vi "CC Main.vi"() -> ()   [LabVIEW 2024]
uses:
  typedefs/CC enum Dither Selection.ctl
  typedefs/CC cluster Hardware Config.ctl
  typedefs/CC cluster Device Index.ctl
  Subsystems/SS cluster Command Queues.ctl
  Subsystems/SS typedef Cmd Queue Reference.ctl
  Subsystems/SS typedef cluster Instrument Command Queue Data.ctl
  hk-channel-class/hk-channel-class/HK Table/HK Table.lvclass
  typedefs/CC cluster System Settings.ctl
  Subsystems/SS cluster Data Queue type.ctl
  Subsystems/Subsystem Class CryoServer/Subsystem CryoServer.lvclass
  C:/Development/rimas/RIMAS/Subsystems/Subsystem Class.lvclass
  Subsystems/Detector/Detector.lvclass
  Subsystems/Subsystem Class Filter Wheel/Subsystem Filter Wheel.lvclass
  Subsystems/Subsystem Class Telescope/Subsystem Telescope.lvclass
  Subsystems/Subsystem Class Focus/Subsystem Class Focus.lvclass
  Subsystems/Subsystem CryoCooler/Subsystem CryoCooler.lvclass
  Subsystems/Subsystem Pressure Monitor/Subsystem Pressure Monitor.lvclass
  Subsystems/Subsystem Class Temp Control/Subsystem Class Temp Control.lvclass
  Subsystems/SS cluster Script Status Queue.ctl
  typedefs/CC cluster Observation.ctl
  Observation Queue/CC enum Observation Status.ctl
  Telescope/CC cluster Telescope Offsets.ctl
  typedefs/CC cluster Observation Dither Options.ctl
  typedefs/CC cluster RA and DEC.ctl
  Telescope/Telescope cluster Rotator.ctl
  library/Activity Log/Activity Log enum Action .ctl
  Subsystems/Subsystem Class.lvclass/Subsystem Class.ctl
  typedefs/CC cluster Script.ctl
  typedefs/CC Script Step.ctl
  typedefs/CC enum Script Action.ctl
  Scripts/CC Rd Wr Script Action.ctl
  typedefs/CC enum Alarm Action.ctl
  Logging/CC enum Current Values Action.ctl
  typedefs/CC cluster Script Status Data.ctl
  Subsystems/SS Read cmd q.vi
  54ac6f3e-f790-48ea-ae38-f3b11f920432.vi
  <vilib>/Utility/error.llb/Trim Whitespace One-Sided.vi
  <vilib>/Utility/TDMS File Viewer/TDMS - File Viewer (NXG Style).vi
  <vilib>/Comparison/Less/Less Functor/Less Functor.lvclass
  <vilib>/regexp/Match Regular Expression.xnode
  Subsystems/Subsystem Class.lvclass
  hk-channel-class/hk-channel-class/HK Item/HK Item.lvclass
  <vilib>/Utility/TDMS File Viewer/NI_TDMS File Viewer.lvlib
panel:
  in  "Tab Control":T1(tab)
  in  "Save As Button":bool
  in  "Load":bool
  in  "Get Image":bool
  in  "DEC dither offset":dbl caption="DEC" format="%.1g"
  in  "RA Dither Offset":dbl caption="RA" format="%.1g"
  in  "Filter 4":u16(ring) caption="Slit" items=["pinhole", "1.2'' long", "2.0''", "1.0''", "0.6''", "open"]
  in  "Filter 3":u16(ring) caption="Aux" items=["open", "ND3", "blank", "H2", "2180", "2190", "Br-g"]
  in  "Priority":i32
  in  "Comment":string
  out "Observation File":string
  in  "Block ID":string
  in  "Images":i32=1 min=1 step=1
  in  "Phase":dbl format="%.1g"
  in  "ROT PA":dbl
  in  "eta":dbl
  in  "xi":dbl
  in  "DEC":string
  in  "RA":string
  in  "Obj Type":T2(ring)
  in  "Obj Name":string
  in  "Observer":string
  in  "Add to Q top":bool
  in  "Add to Q":bool
  out "Current DEC":string
  out "Current RA":string
  in  "Replace":bool
  in  "Add Obs Row":bool
  in  "Generate Script":bool
  in  "Save Obs List":bool
  in  "Radius":dbl format="%.1g"
  in  "Int Time":dbl format="%.1g"
  in  "Spots":i32=1 min=1 step=1
  in  "Dither":T3
  in  "Filter 2":u16(ring) caption="FW HK" items=["Grism", "Open", "Vph30", "Vph300", "H", "K"]
  in  "Filter 1":u16(ring) caption="FW YJ" items=["Grism", "Open", "Vph30", "Vph300", "J", "Y"]
  in  "Observation List":i32[](listbox)
  in  "Edit FITS Hdr":bool
  in  "Log 2":bool caption="Log"
  in  "Log":bool
  in  "Export Cryo Data":bool
  out "XY Graph":cluster{timestamp[], dbl[]}[](graph)
  in  "Plot":bool
  in  "Channels":i32[](listbox)
  in  "Open Log":bool
  in  "Note for Log":string
  in  "Send":bool
  in  "Close":bool
  in  "Image Type":u16(ring) items=["raw", "res"]
  in  "Recent Images":i32(listbox)
  out "Status":string
  out "Progress":u8(slide) scale=0.0..100.0
  out "Current File":string
  in  "Data Folder":path
  in  "Clear Alarms":bool
  out "Temp":bool
  out "Cryo Alarm":bool
  out "Pressure Alarm":bool
  out "Telescope Alarm":bool
  out "FW Alarm":bool
  out "Detector Alarm":bool
  out "Alarm Message":string
  out "Alarm Status":bool
  in  "Add offsets":bool
  out "offset (\")":dbl[](array[numeric]) format="%#_3g"
  out "Thumbnail":sgl[][](graph)
  in  "zoom size":i32=20
  out "Zoom":sgl[][](graph)
  out "Console":string
  in  "Tab Control 2":enum32{"Observation Queue", "Slice"}(tab)
  out "Waveform Graph":cluster{"image":sgl[]}[](graph)
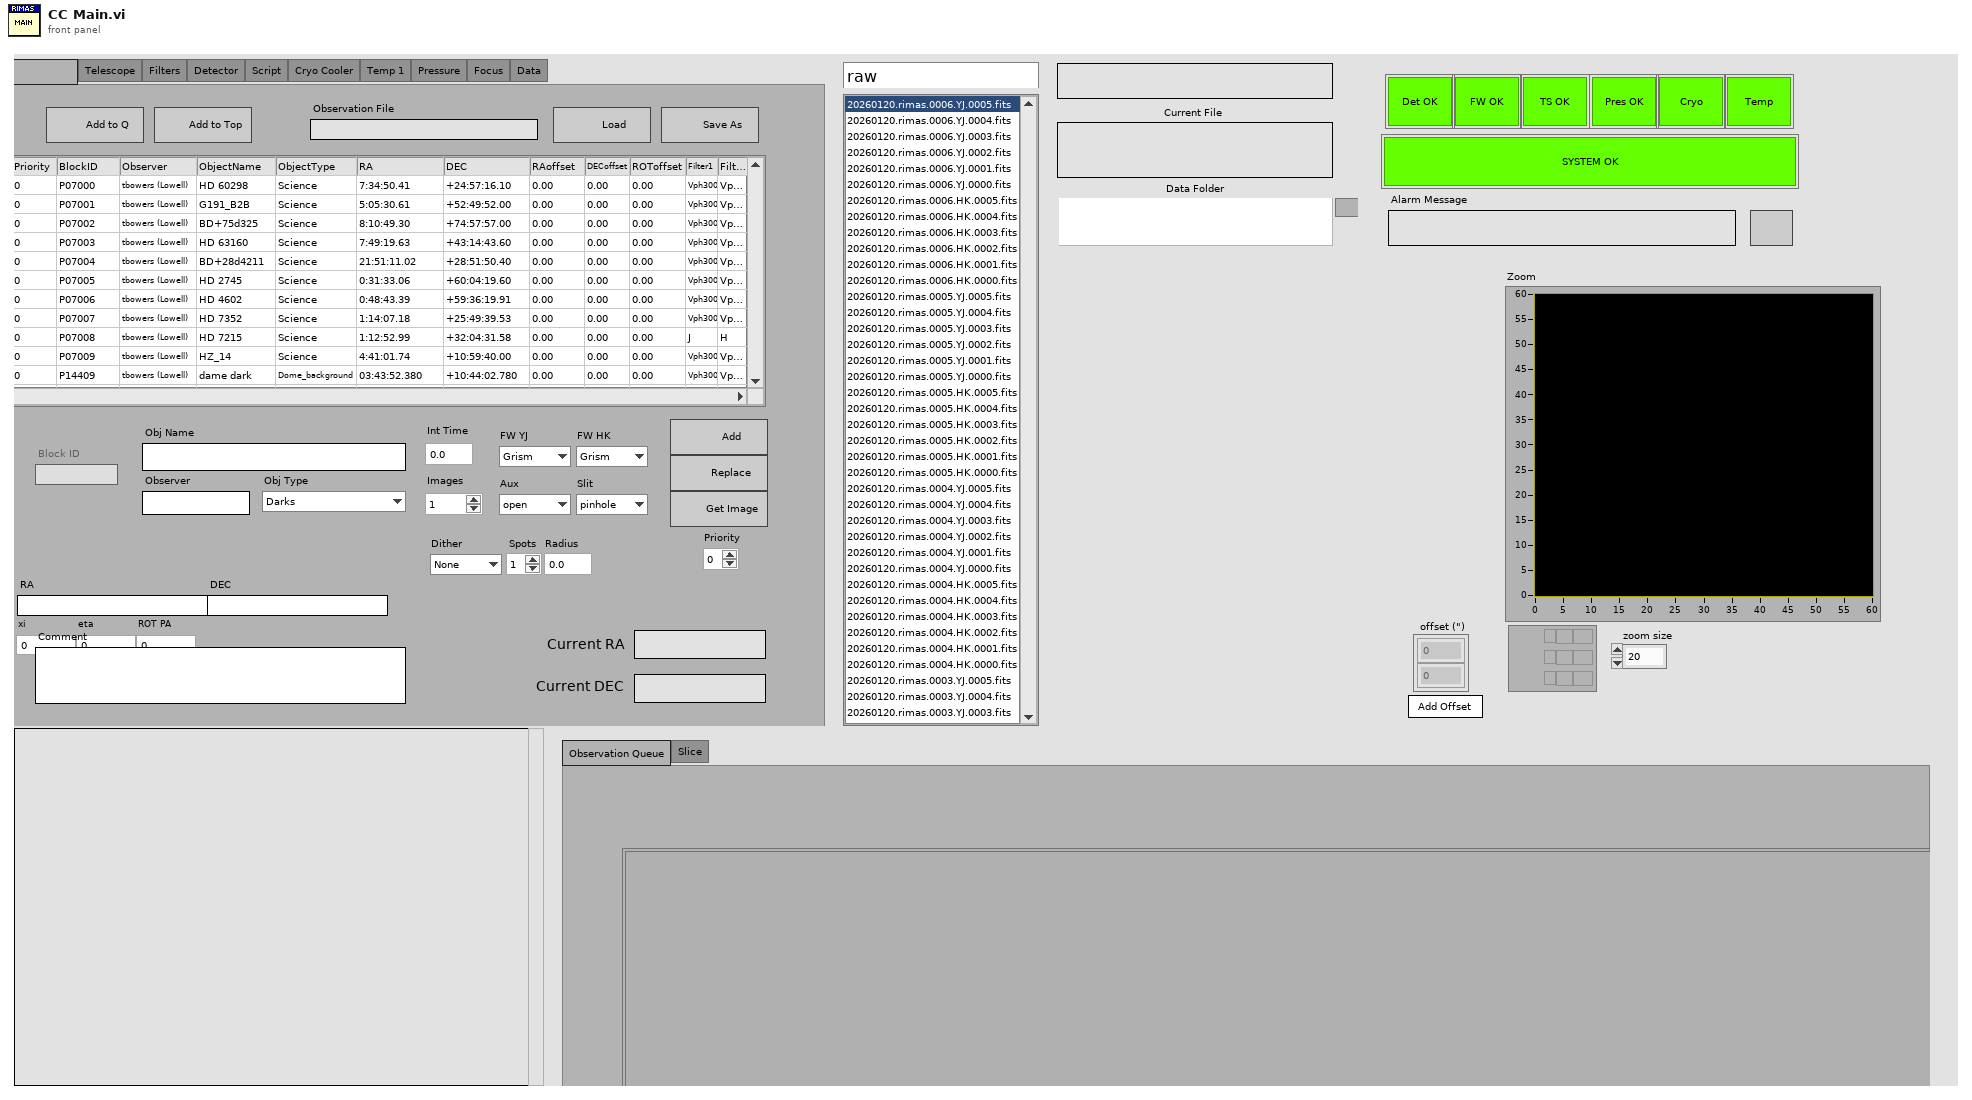
[diagram p1: front panel]
types:
  T1 = enum32{"Observations", "Telescope", "Filters", "Detector", "Script", "Temperatures", "Cryo Cooler", "Temp 1", "Temp 2", "Temp 3", "Pressure", "Focus", "Data"}
  T2 = enum16{"Darks", "Dome_flat", "Sky_flat", "Comparison_lamp", "Comparison_sky", "Dome_background", "Science", "Science_crowded", "Science_extended", "a0v", "Standard", "Tel_focus", "Inst_focus", "Test"}
  T3 = typedef "CC enum Dither Selection.ctl" = enum16{"None", "Circle", "Random", "ABBA", "OnOff"}
  T4 = enum32{"invalid app kind", "Development System", "Run Time System", "Student Edition", "Embedded LabVIEW", "Evaluation", "Custom"}
  T5 = typedef "CC cluster Hardware Config.ctl" = cluster{"Installed Hardware":T6[]}
  T6 = typedef "CC cluster Device Index.ctl" = cluster{"Device Type Name":string, "Curr Device Name":string, "All Instances":string[]}
  T7 = typedef "SS cluster Command Queues.ctl" = cluster{"Telescope Q":T8, "Filter Wheel Q":T8, "Script Q":T8, "CryoServer Q":T8, "Detector Q":T8, "Focus Q":T8, "Temp Ctl 1":T8, "Temp Ctl 2":T8, "Temp Ctl 3":T8, "CryoCooler Q":T8, "Pressure Q":T8}
  T8 = typedef "SS typedef Cmd Queue Reference.ctl" = refnum<queue>
  T9 = typedef "CC cluster System Settings.ctl" = cluster{"HK Table Name":string, "Images Folder":path, "Obs File":path}
  T10 = typedef "CC cluster Observation.ctl" = cluster{"Priority":i32, "ID":string, "Observer":string, "Obj Name":string, "Obj Type":string, "RA and DEC String":cluster{"RA":string, "DEC":string}, "Filters":string[], "Integration Time":dbl, "Observation Status":T11, "Offsets":T12, "Images":i32, "Dither Options":T13, "Comment 1":string, "Comment 2":string, "Rotator":T15}
  T11 = typedef "CC enum Observation Status.ctl" = enum16{"Ready", "Running", "Done", "Error"}
  T12 = typedef "CC cluster Telescope Offsets.ctl" = cluster{"xi":dbl, "eta":dbl, "Offset Type":enum16{"SIMPLE", "TPLANE", "PA"}}
  T13 = typedef "CC cluster Observation Dither Options.ctl" = cluster{"Dither":T3, "Dither Radius":dbl, "Dither Points":i32, "Dither Phase":dbl, "B Offset":T14}
  T14 = typedef "CC cluster RA and DEC.ctl" = cluster{"RA":dbl, "DEC":dbl}
  T15 = typedef "Telescope cluster Rotator.ctl" = cluster{"Frame":enum16{"Target", "Fixed"}, "PA":dbl}
  T16 = cluster{"state":refnum<user-event>, "Hardware":T5, "error":errorcluster, "Cmd Qs":T7, "HK Channels":refnum<class "HK Table.lvclass">, "System Settings":T9, "Data Q":refnum<queue>, "file path":path, "SS":cluster{"CryoServer":refnum<class "Subsystem CryoServer.lvclass">, "Detector":refnum<class "Detector.lvclass">, "Filter Wheel":refnum<class "Subsystem Filter Wheel.lvclass">, "Telescope":refnum<class "Subsystem Telescope.lvclass">, "Focus":refnum<class "Subsystem Class Focus.lvclass">, "CryoCooler":refnum<class "Subsystem CryoCooler.lvclass">, "Pressure":refnum<class "Subsystem Pressure Monitor.lvclass">, "Temp Ctl 1":refnum<class "Subsystem Class Temp Control.lvclass">, "Temp Ctl 2":refnum<class "Subsystem Class Temp Control.lvclass">, "Temp Ctl 3":refnum<class "Subsystem Class Temp Control.lvclass">}, "Script Status Q":refnum<queue>, "Status Data":variant, "curr image":path, "image":sgl[][], "Application:Kind":enum32{"invalid app kind", "Development System", "Run Time System", "Student Edition", "Embedded LabVIEW", "Evaluation", "Custom"}, "Observation List":T10[], "Viewer Ref":refnum<vi>, "Quad Viewer Ref":refnum<vi>, "Obs Queue":refnum<queue>, "Queue vi ref":refnum<vi>, "Script Running":bool, "Wheel Ref":refnum<vi>[], "Observation":T10, "alarm disable":bool, "image types":map{string, path}}
  T17 = typedef "SS cluster Data Queue type.ctl" = cluster{"Source":string, "Type":string, "Data":variant}
  T18 = typedef "Activity Log enum Action .ctl" = enum16{"Add Entry", "Get Log", "Restore From Disk", "Save to Disk", "Init"}
  T19 = typedef "SS typedef cluster Instrument Command Queue Data.ctl" = cluster{"Cmd":string, "Parameters":variant}
  T20 = enum8{"Enabled", "Disabled", "Disabled and Grayed Out"}
  T21 = typedef "CC Rd Wr Script Action.ctl" = enum16{"Read", "Write", "List", "Delete"}
  T22 = typedef "CC cluster Script.ctl" = cluster{"Name":string, "Script":T23[]}
  T23 = typedef "CC Script Step.ctl" = cluster{"Action":T24, "Data":variant}
  T24 = typedef "CC enum Script Action.ctl" = enum16{"Noop", "Define Object", "Define Exposure", "Define Dithering", "Acquire Images", "Set Filter Wheel", "Telescope Home", "Telescope Move", "Telescope RA DEC", "Focus Move Relative", "Focus Move Absolute", "Focus Set Home", "Macro", "Pause", "Ask User", "Define Random Dither", "CmdLine", "Outlet"}
  T25 = typedef "CC enum Alarm Action.ctl" = enum16{"Init", "Add Alarm", "Get Alarms", "Clear Alarm", "Clear All Alarms"}
  T26 = typedef "CC enum Current Values Action.ctl" = enum16{"Init", "Write Item", "Write Array", "Read Item", "Read Array", "Read All", "Add Channels", "New File", "Add Message", "Get Current Values", "Close"}
  T27 = typedef "CC cluster Script Status Data.ctl" = cluster{"Time":timestamp, "Running":bool, "Step":i32, "Script Name":string, "Step Name":string}
  T28 = typedef "SS cluster Script Status Queue.ctl" = cluster{"Msg":string, "Data":variant}
  T29 = typedef "CC cluster Script Panel Defaults.ctl" = cluster{"Script Name":string, "Script Path":path}
  T30 = typedef "CC cluster Alarm Data.ctl" = cluster{"Measured Value":dbl, "Alarm Low":dbl, "Alarm High":dbl, "Message":string, "Source":string}
  T31 = typedef "SS cluster New Image Data.ctl" = cluster{"Frame number":i32, "Detector #":u16, "FITS file":path, "File size":i64, "Image Type":string}
  T32 = typedef "LVCursorListTypeDef.ctl" = cluster{"Name":string, "Color":u32, "Style":u8, "Point Style":u8, "Name Visible":bool, "Allow Drag":bool, "Cursor Mode":u32, "Plot":i32, "Index":i32, "Position":cluster{"X":dbl, "Y":dbl}, "X Scale":u32, "Y Scale":u32, "Watch Plots":i32[], "Watch All Plots":bool, "Plot Area":i32, "Label Offset":cluster{"X":dbl, "Y":dbl}}[]
  T33 = cluster{"Name":string, "Color":u32, "Style":u8, "Point Style":u8, "Name Visible":bool, "Allow Drag":bool, "Cursor Mode":u32, "Plot":i32, "Index":i32, "Position":cluster{"X":dbl, "Y":dbl}, "X Scale":u32, "Y Scale":u32, "Watch Plots":i32[], "Watch All Plots":bool, "Plot Area":i32, "Label Offset":cluster{"X":dbl, "Y":dbl}}
  T34 = cluster{"CryoServer":refnum<class "Subsystem CryoServer.lvclass">, "Detector":refnum<class "Detector.lvclass">, "Filter Wheel":refnum<class "Subsystem Filter Wheel.lvclass">, "Telescope":refnum<class "Subsystem Telescope.lvclass">, "Focus":refnum<class "Subsystem Class Focus.lvclass">, "CryoCooler":refnum<class "Subsystem CryoCooler.lvclass">, "Pressure":refnum<class "Subsystem Pressure Monitor.lvclass">, "Temp Ctl 1":refnum<class "Subsystem Class Temp Control.lvclass">, "Temp Ctl 2":refnum<class "Subsystem Class Temp Control.lvclass">, "Temp Ctl 3":refnum<class "Subsystem Class Temp Control.lvclass">}
  T35 = typedef "LVPoint32TypeDef.ctl" = cluster{"Horizontal":i32, "Vertical":i32}
  T36 = typedef "LVRowAndColumnTypeDef.ctl" = cluster{"Row":i32, "Column":i32}
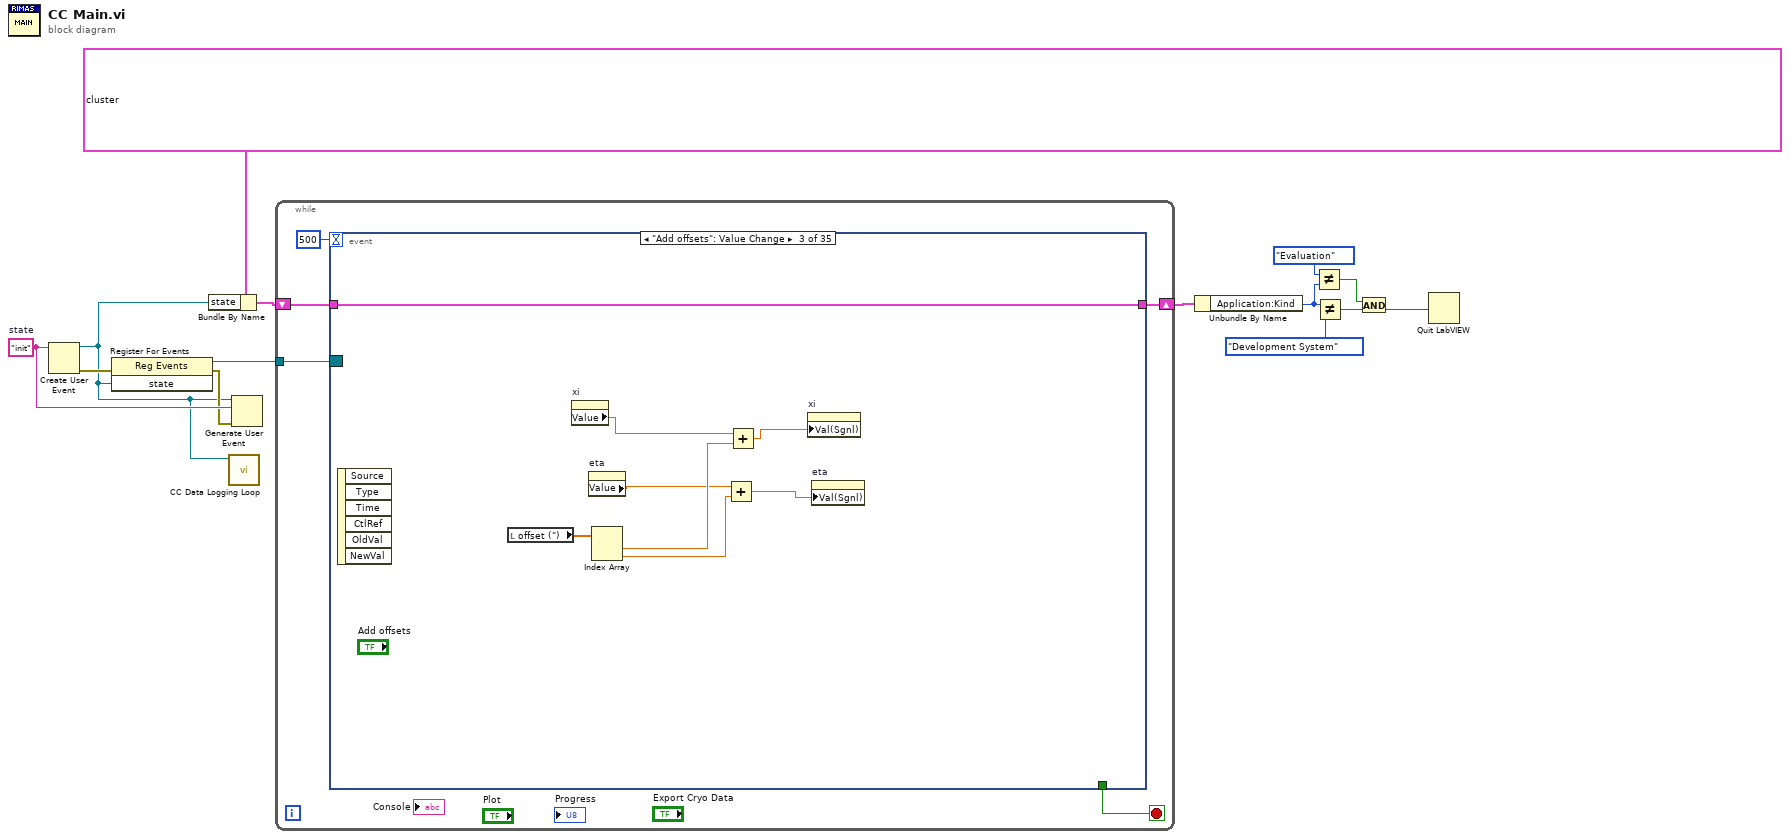
[diagram p0: block diagram]
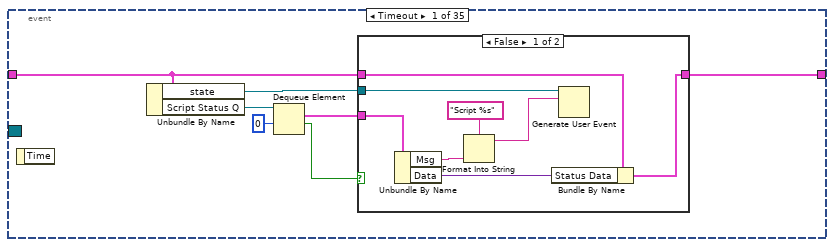
[diagram p2: hidden frame]
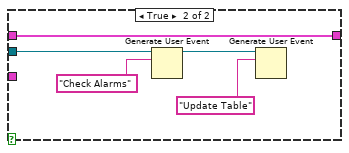
[diagram p3: hidden frame]
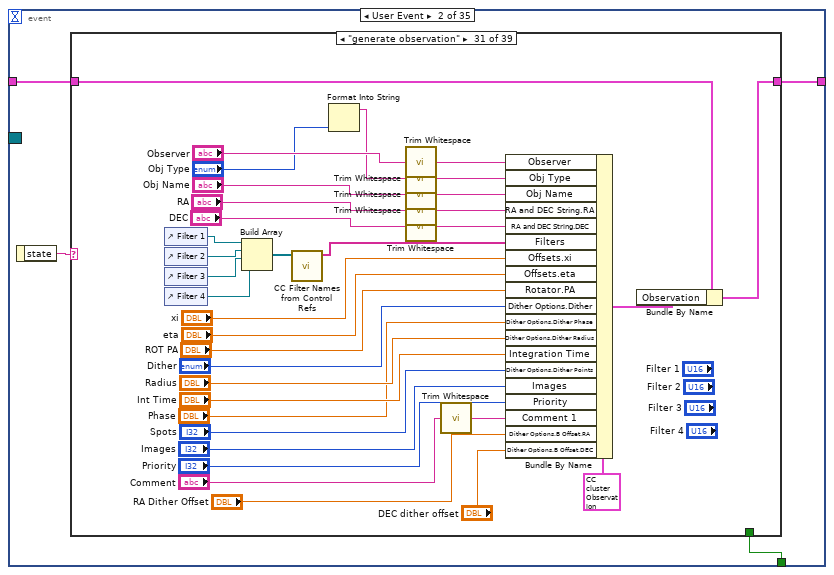
[diagram p4: hidden frame]
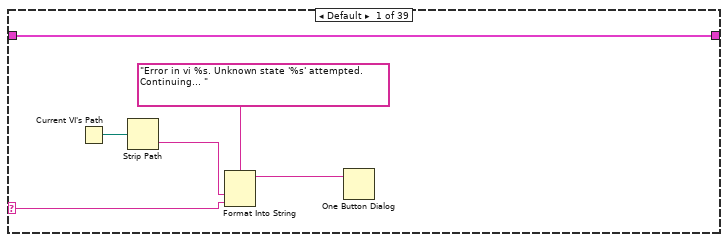
[diagram p5: hidden frame]
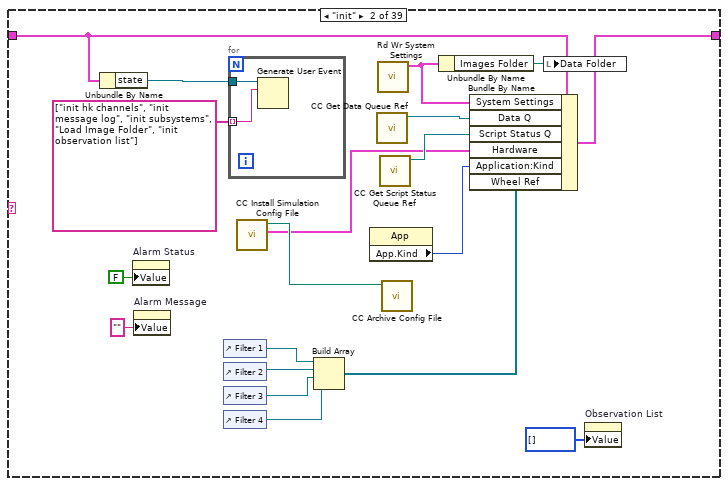
[diagram p6: hidden frame]
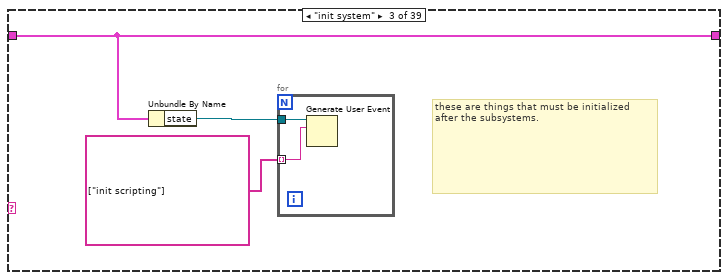
[diagram p7: hidden frame]
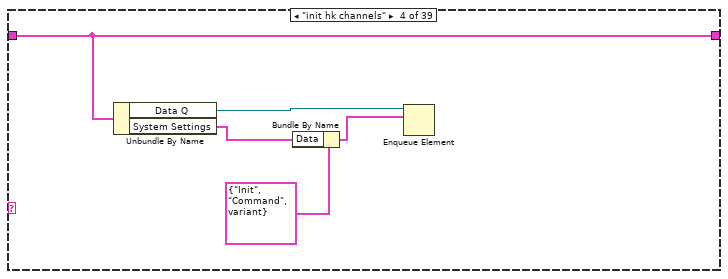
[diagram p8: hidden frame]
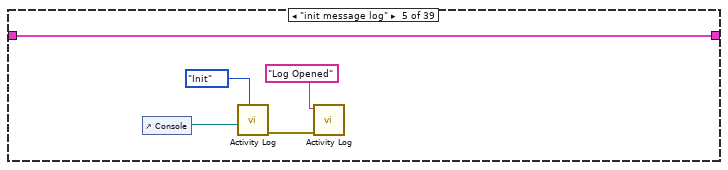
[diagram p9: hidden frame]
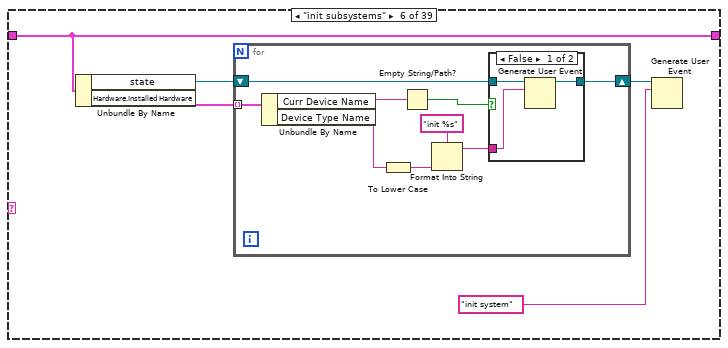
[diagram p10: hidden frame]
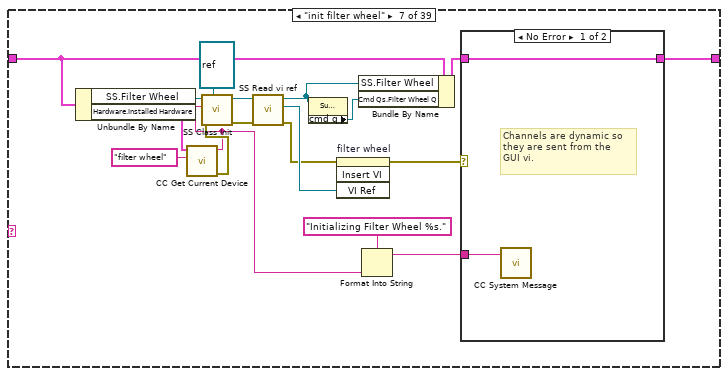
[diagram p12: hidden frame]
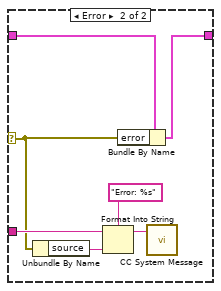
[diagram p13: hidden frame]
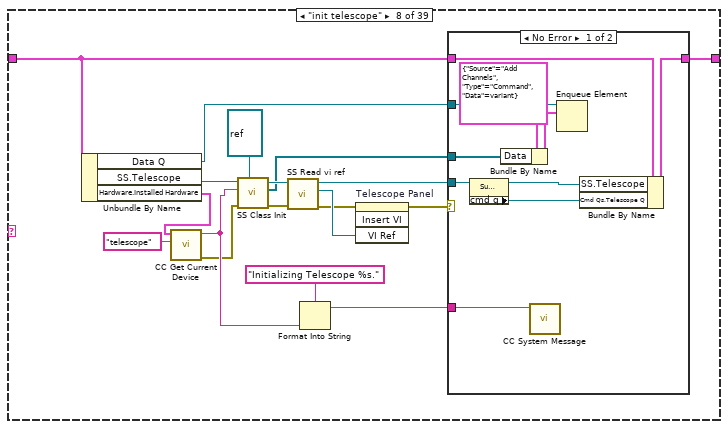
[diagram p14: hidden frame]
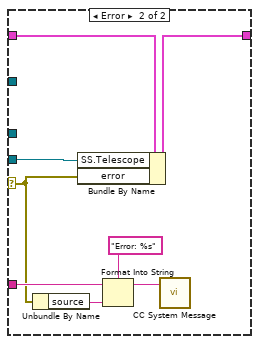
[diagram p15: hidden frame]
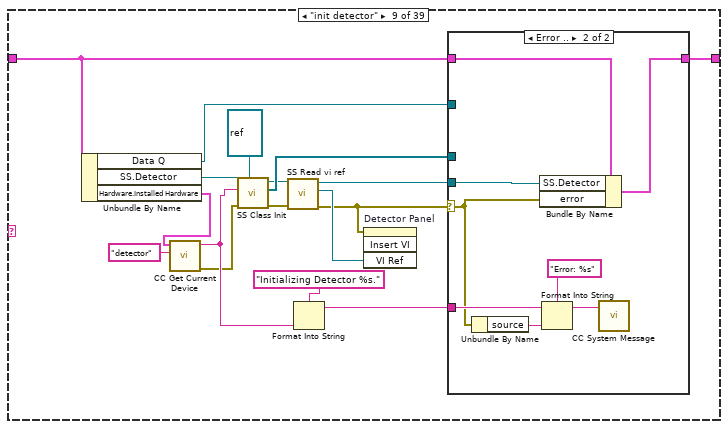
[diagram p16: hidden frame]
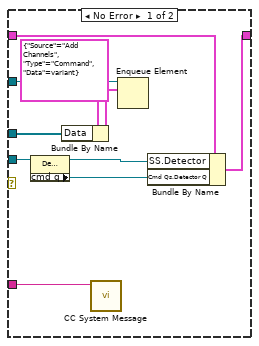
[diagram p17: hidden frame]
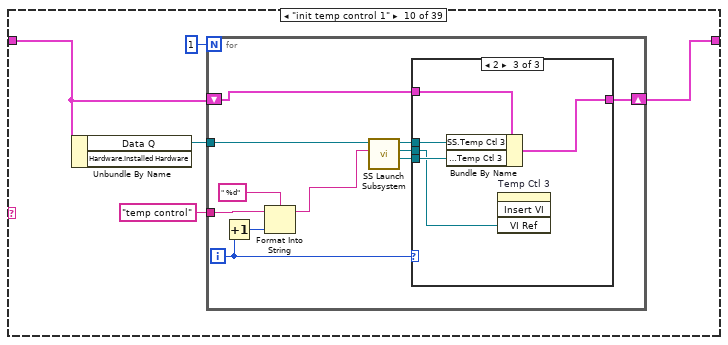
[diagram p18: hidden frame]
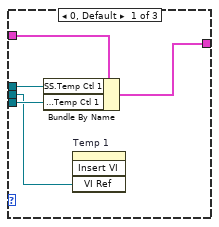
[diagram p19: hidden frame]
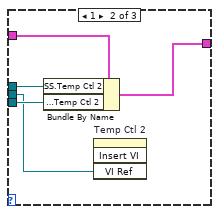
[diagram p20: hidden frame]
diagram:
  w11 = "init"  # state
  n1 = Create User Event(user event datatype=w11) -> (user event=w8:refnum<user-event>, error out=w9:errorcluster)  [unwired: 1 in]
  n2 = register-events(error in=w9, w8) -> (reference out=w12:refnum<event-registration>, error out=w10:errorcluster)  [unwired: 1 in]
  n3 = Bundle By Name(cluster=T16 {"state"=refnum, "Hardware"={"Installed Hardware"=[]}, "error"={"status"=FALSE, "code"=0, "source"=""}, "Cmd Qs"={"Telescope Q"=refnum, "Filter Wheel Q"=refnum, "Script Q"=refnum, "CryoServer Q"=refnum, "Detector Q"=refnum, "Focus Q"=refnum, "Temp Ctl 1"=refnum, "Temp Ctl 2"=refnum, "Temp Ctl 3"=refnum, "CryoCooler Q"=refnum, "Pressure Q"=refnum}, "HK Channels"=refnum, "System Settings"={"HK Table Name"="", "Images Folder"=path "", "Obs File"=path ""}, "Data Q"=refnum, "file path"=path "", "SS"={"CryoServer"=refnum, "Detector"=refnum, "Filter Wheel"=refnum, "Telescope"=refnum, "Focus"=refnum, "CryoCooler"=refnum, "Pressure"=refnum, "Temp Ctl 1"=refnum, "Temp Ctl 2"=refnum, "Temp Ctl 3"=refnum}, "Script Status Q"=refnum, "Status Data"=variant, "curr image"=path "", "image"=[], "Application:Kind"=enum."invalid app kind", "Observation List"=[], "Viewer Ref"=refnum, "Quad Viewer Ref"=refnum, "Obs Queue"=refnum, "Queue vi ref"=refnum, "Script Running"=FALSE, "Wheel Ref"=[], "Observation"={"Priority"=0, "ID"="", "Observer"="", "Obj Name"="", "Obj Type"="", "RA and DEC String"={"RA"="12:34:56.789", "DEC"="010:11:12.013"}, "Filters"=[], "Integration Time"=0.0, "Observation Status"=enum."Ready", "Offsets"={"xi"=0.0, "eta"=0.0, "Offset Type"=enum."SIMPLE"}, "Images"=0, "Dither Options"={"Dither"=enum."None", "Dither Radius"=0.0, "Dither Points"=0, "Dither Phase"=0.0, "B Offset"={"RA"=0.0, "DEC"=0.0}}, "Comment 1"="", "Comment 2"="", "Rotator"={"Frame"=enum."Target", "PA"=0.0}}, "alarm disable"=FALSE, "image types"={}}, "state"=w8) -> (w13:T16)
  n4 = call "CC Data Logging Loop.vi"("user event"=w8) -> ()  [unwired: 11 in]
  n5 = Generate User Event(user event=w8, event data cluster=w11, error in=w10) -> ()  [unwired: 1 in, 2 out]
  n6 = while {
    tunnel: w12 -> [w19]
    shift-right: [w17] -> w7
    shift-left: w13 -> [w18]
    stop <- w16 stop-if-true
    n7 = event shown="[2] \"Add offsets\": Value Change" {
      selector: w19 -> [_ _ _ _ _ _ _ _ _ _ _ _ _ _ _ _ _ _ _ _ _ _ _ _ _ _ _ _ _ _ _ _ _ _ _]
      dyn-events: _ -> [_ _ _ _ _ _ _ _ _ _ _ _ _ _ _ _ _ _ _ _ _ _ _ _ _ _ _ _ _ _ _ _ _ _ _]
      timeout: 500 -> [_ _ _ _ _ _ _ _ _ _ _ _ _ _ _ _ _ _ _ _ _ _ _ _ _ _ _ _ _ _ _ _ _ _ _]
      tunnel: w18 -> [w24 w42 w809 w812 w878 w881 w917 w919 w924 w954 w985 w991 w1011 w1019 w1022 w1027 w1033 w1039 w1042 w1044 w1051 w1189 w1202 w1219 w1222 w1225 w1227 w1230 w1236 w1237 w1245 w1259 w1263 w1270 w1276]
      tunnel: [w21 w41 w809 w811 w878 w881 w917 w919 w926 w954 w985 w992 w1011 w1019 w1022 w1027 w1033 w1039 w1042 w1044 w1052 w1189 w1204 w1219 w1222 w1225 w1227 w1230 w1236 w1237 w1241 w1259 w1263 w1267 w1276] -> w17
      tunnel: [_ w40 _ _ _ _ _ _ _ _ _ _ _ _ _ _ _ _ _ _ _ _ _ _ _ _ _ _ FALSE ("Close") _ _ _ _ _ _] -> w16
      event Timeout {
        n8 = event-data() -> ()  [unwired: 1 in, 1 out]
        n9 = Unbundle By Name(w24) -> ("state"=w23:refnum<user-event>, "Script Status Q"=w26:refnum<queue>)
        n10 = Dequeue Element(queue=w26, timeout in ms (-1)=0) -> (element=w22:T28, timed out?=w25:bool)  [unwired: 1 in, 2 out]
        n11 = case shown="False" w25 {
          tunnel: w24 -> [w29 w39]
          tunnel: w23 -> [w34 w38]
          tunnel: w22 -> [w33 _]
          tunnel: [w27 w39] -> w21
          frame False {
            n12 = Unbundle By Name(w33) -> ("Msg"=w31:string, "Data"=w28:variant)
            n13 = Format Into String(format string="Script %s", w31) -> (resulting string=w30:string)  [unwired: 2 in, 1 out]
            n14 = Bundle By Name(cluster=w29, "Status Data"=w28) -> (w27:T16)
            n15 = Generate User Event(user event=w34, event data cluster=w30) -> ()  [unwired: 2 in, 2 out]
          }
          frame True {
            n16 = Generate User Event(user event=w38, event data cluster="Check Alarms" ("event data")) -> (user event out=w36:refnum<user-event>)  [unwired: 2 in, 1 out]
            n17 = Generate User Event(user event=w36, event data cluster="Update Table" ("event data")) -> ()  [unwired: 2 in, 2 out]
          }
        }
      }
      event User Event {
        n18 = event-data() -> ("state"=w43:string)  [unwired: 1 in]
        n19 = case shown="\"generate observation\"" w43 {
          selector: w43 -> [w48 _ _ _ _ _ _ _ _ _ _ _ _ _ _ _ _ _ _ _ _ _ _ _ _ _ _ _ _ _ _ _ _ _ _ _ _ _ _]
          tunnel: w42 -> [w44 w65 w72 w76 w85 w90 w114 w144 w181 w204 w233 w244 w276 w307 w342 w364 w395 w404 w419 w437 w446 w453 w478 w497 w542 w568 w598 w616 w656 w663 w675 w706 w713 w721 w725 w770 w773 w782 w792]
          tunnel: [w44 w66 w72 w76 w85 w90 w115 w145 w182 w203 w233 w245 w277 w308 w343 w365 w396 w405 w418 w437 w446 w453 w478 w498 w542 w568 w599 w617 w656 w664 w676 w706 w713 w722 w726 w770 w773 w782 w792] -> w41
          tunnel: [_ _ _ _ _ _ _ _ _ _ _ _ _ _ _ _ _ _ _ _ _ _ _ _ _ _ _ _ _ _ _ _ _ _ _ _ _ FALSE TRUE] -> w40
          frame Default {
            n20 = Current VI's Path() -> (path=w47:path)
            n21 = Strip Path(path=w47) -> (name=w46:string)  [unwired: 1 out]
            n22 = Format Into String(format string="Error in vi %s. Unknown state '%s' attempted. Continuing... ", w46, w48) -> (resulting string=w45:string)  [unwired: 2 in, 1 out]
            n23 = One Button Dialog(message=w45) -> ()  [unwired: 1 in, 1 out]
          }
          frame "init" {
            n24 = Unbundle By Name(w65) -> ("state"=w68:refnum<user-event>)
            n25 = property on="Alarm Status" class="Bool (strict)"("Value"=FALSE ("Alarm Status")) -> ()  [unwired: 2 in, 2 out]
            n26 = property on="Alarm Message" class="Str"("Value"="" ("Alarm Message")) -> ()  [unwired: 2 in, 2 out]
            n27 = control-ref of="Filter 1"() -> (w56:refnum<vi>)
            n28 = control-ref of="Filter 2"() -> (w55:refnum<vi>)
            n29 = control-ref of="Filter 3"() -> (w54:refnum<vi>)
            n30 = control-ref of="Filter 4"() -> (w53:refnum<vi>)
            n31 = for {
              tunnel: w68 -> [w70]
              tunnel: string[] ["init hk channels", "init message log", "init subsystems", "Load Image Folder", "init observation list"] -> [w69] mode=indexing
              n32 = Generate User Event(user event=w70, event data cluster=w69) -> ()  [unwired: 2 in, 2 out]
            }
            n33 = call "CC Install Simulation Config File.vi"() -> ("Hardware Config out"=w50:T5, "new path"=w51:path)  [unwired: 10 in]
            n34 = Build Array(w56, w55, w54, w53) -> (w52:refnum<vi>[])
            n35 = property class="App"() -> ("App.Kind"=w60:T4)  [unwired: 2 in, 2 out]
            n36 = call "CC Get Data Queue Ref.vi"() -> ("Data Q"=w64:refnum<queue>)  [unwired: 10 in, 1 out]
            n37 = call "Rd Wr System Settings.vi"() -> ("System Settings out"=w62:T9)  [unwired: 10 in, 1 out]
            n38 = call "CC Get Script Status Queue Ref.vi"() -> ("Script Status Q"=w63:refnum<queue>)  [unwired: 10 in, 1 out]
            n39 = call "CC Archive Config File.vi"("config file"=w51) -> ()  [unwired: 10 in, 1 out]
            n40 = Unbundle By Name(w62) -> ("Images Folder"=w61:path)
            n41 = Bundle By Name(cluster=w65, "System Settings"=w62, "Data Q"=w64, "Script Status Q"=w63, "Hardware"=w50, "Application:Kind"=w60, "Wheel Ref"=w52) -> (w66:T16)
            n42 = local write "Data Folder"(w61) -> ()
            n43 = property on="Observation List" class="MCListbox (strict)"("Value"=i32[] [] ("Observation List")) -> ()  [unwired: 2 in, 2 out]
          }
          frame "init system" {
            # "these are things that must be initialized after the subsystems."
            n44 = Unbundle By Name(w72) -> ("state"=w73:refnum<user-event>)
            n45 = for {
              tunnel: w73 -> [w75]
              tunnel: string[] ["init scripting"] -> [w74] mode=indexing
              n46 = Generate User Event(user event=w75, event data cluster=w74) -> ()  [unwired: 2 in, 2 out]
            }
          }
          frame "init hk channels" {
            n47 = Unbundle By Name(w76) -> ("Data Q"=w80:refnum<queue>, "System Settings"=w78:T9)
            n48 = Bundle By Name(cluster=T17 {"Source"="Init", "Type"="Command", "Data"=variant} ("element"), "Data"=w78) -> (w77:T17)
            n49 = Enqueue Element(queue=w80, element=w77) -> ()  [unwired: 2 in, 3 out]
          }
          frame "init message log" {
            n50 = control-ref of="Console"() -> (w83:refnum<vi>)
            n51 = call "Activity Log.vi"("Action"=Activity_Log_enum_Action_."Init", "string ref"=w83) -> ("Error Out"=w82:errorcluster)  [unwired: 8 in, 1 out]
            n52 = call "Activity Log.vi"("Error In"=w82, "Message Log Entry"="Log Opened") -> ()  [unwired: 8 in, 2 out]
          }
          frame "init subsystems" {
            n53 = Unbundle By Name(w90) -> ("state"=w89:refnum<user-event>, "Hardware.Installed Hardware"=w88:T6[])
            n54 = for {
              tunnel: w88 -> [w97] mode=indexing
              shift-right: [w91] -> w87
              shift-left: w89 -> [w98]
              n55 = Unbundle By Name(w97) -> ("Curr Device Name"=w93:string, "Device Type Name"=w92:string)
              n56 = To Lower Case(string=w92) -> (all lower case string=w94:string)
              n57 = Empty String/Path?(string/path=w93) -> (empty?=w99:bool)
              n58 = Format Into String(format string="init %s", w94) -> (resulting string=w96:string)  [unwired: 2 in, 1 out]
              n59 = case shown="False" w99 {
                tunnel: w98 -> [w102 w103]
                tunnel: w96 -> [w101 _]
                tunnel: [w100 w103] -> w91
                frame False {
                  n60 = Generate User Event(user event=w102, event data cluster=w101) -> (user event out=w100:refnum<user-event>)  [unwired: 2 in, 1 out]
                }
                frame True {
                }
              }
            }
            n61 = Generate User Event(user event=w87, event data cluster="init system" ("format string")) -> ()  [unwired: 2 in, 2 out]
          }
          frame "init filter wheel" {
            n62 = Unbundle By Name(w114) -> ("SS.Filter Wheel"=w113:refnum<class "Subsystem Filter Wheel.lvclass">, "Hardware.Installed Hardware"=w107:T6[])
            n63 = call "CC Get Current Device.vi"("Device Type Name"="filter wheel", "Hardware.Installed Hardware"=w107) -> ("error out"=w105:errorcluster, "Curr Device Name"=w104:string)  [unwired: 7 in, 1 out]
            n64 = call-dynamic "SS Class Init.vi"("VI Refnum"=refnum<vi> refnum, "error in (no error)"=w105, "Device"=w104, "Subsystem Filter Wheel in"=w113) -> ("error out"=w109:errorcluster, "Subsystem Filter Wheel out"=w112:refnum<class "Subsystem Filter Wheel.lvclass">)  [unwired: 5 in, 1 out]
            n65 = call "SS Read vi ref.vi"("error in (no error)"=w109, "Subsystem Class in"=w112) -> ("error out"=w120:errorcluster, "vi ref"=w121:refnum<vi>, "Subsystem Class out"=w111:refnum<class "Subsystem Filter Wheel.lvclass">)  [unwired: 7 in]
            n66 = property class="Subsystem Filter Wheel.lvclass"(reference=w111) -> ("cmd q"=w110:T8)  [unwired: 1 in, 2 out]
            n67 = invoke on="filter wheel" class="SubPnl" method="Insert VI"(error in=w120, "VI Ref"=w121) -> (error out=w118:errorcluster)  [unwired: 2 in, 3 out]
            n68 = Bundle By Name(cluster=w114, "SS.Filter Wheel"=w111, "Cmd Qs.Filter Wheel Q"=w110) -> (w116:T16)
            n69 = Format Into String(format string="Initializing Filter Wheel %s.", w104) -> (resulting string=w117:string)  [unwired: 2 in, 1 out]
            n70 = case shown="No Error" w118 {
              selector: w118 -> [_ w126]
              tunnel: w117 -> [w123 w127]
              tunnel: w116 -> [w122 w130]
              tunnel: [w122 w129] -> w115
              frame No Error {
                # "Channels are dynamic so\nthey are sent from the \nGUI vi."
                n71 = call "CC System Message.vi"("Message"=w123) -> ()  [unwired: 10 in, 1 out]
              }
              frame Error {
                n72 = Unbundle By Name(w126) -> ("source"=w125:string)
                n73 = Format Into String(format string="Error: %s", initial string=w127, w125) -> (resulting string=w124:string)  [unwired: 1 in, 1 out]
                n74 = Bundle By Name(cluster=w130, "error"=w126) -> (w129:T16)
                n75 = call "CC System Message.vi"("Message"=w124) -> ()  [unwired: 10 in, 1 out]
              }
            }
          }
          frame "init telescope" {
            n76 = Unbundle By Name(w144) -> ("Data Q"=w136:refnum<queue>, "SS.Telescope"=w148:refnum<class "Subsystem Telescope.lvclass">, "Hardware.Installed Hardware"=w133:T6[])
            n77 = call "CC Get Current Device.vi"("Device Type Name"="telescope", "Hardware.Installed Hardware"=w133) -> ("error out"=w131:errorcluster, "Curr Device Name"=w132:string)  [unwired: 7 in, 1 out]
            n78 = call-dynamic "SS Class Init.vi"("VI Refnum"=refnum<vi> refnum, "error in (no error)"=w131, "Device"=w132, "Telescope in"=w148) -> ("error out"=w146:errorcluster, "Channel List"=w137:refnum<class "HK Item.lvclass">[], "Telescope out"=w147:refnum<class "Subsystem Telescope.lvclass">)  [unwired: 5 in]
            n79 = call "SS Read vi ref.vi"("error in (no error)"=w146, "Subsystem Class in"=w147) -> ("error out"=w139:errorcluster, "vi ref"=w140:refnum<vi>, "Subsystem Class out"=w141:refnum<class "Subsystem Telescope.lvclass">)  [unwired: 7 in]
            n80 = Format Into String(format string="Initializing Telescope %s.", w132) -> (resulting string=w142:string)  [unwired: 2 in, 1 out]
            n81 = invoke on="Telescope Panel" class="SubPnl" method="Insert VI"(error in=w139, "VI Ref"=w140) -> (error out=w138:errorcluster)  [unwired: 2 in, 3 out]
            n82 = case shown="No Error" w138 {
              selector: w138 -> [_ w162]
              tunnel: w142 -> [w149 w163]
              tunnel: w144 -> [w155 w166]
              tunnel: [w156 w165] -> w145
              tunnel: w141 -> [w158 w160]
              tunnel: w137 -> [w151 _]
              tunnel: w136 -> [w153 _]
              frame No Error {
                n83 = property class="Subsystem Telescope.lvclass"(reference=w158) -> (reference out=w154:refnum<class "Subsystem Telescope.lvclass">, "cmd q"=w157:T8)  [unwired: 1 in, 1 out]
                n84 = Bundle By Name(cluster=T17 {"Source"="Add Channels", "Type"="Command", "Data"=variant} ("element"), "Data"=w151) -> (w150:T17)
                n85 = call "CC System Message.vi"("Message"=w149) -> ()  [unwired: 10 in, 1 out]
                n86 = Enqueue Element(queue=w153, element=w150) -> ()  [unwired: 2 in, 3 out]
                n87 = Bundle By Name(cluster=w155, "SS.Telescope"=w154, "Cmd Qs.Telescope Q"=w157) -> (w156:T16)
              }
              frame Error {
                n88 = Unbundle By Name(w162) -> ("source"=w161:string)
                n89 = Bundle By Name(cluster=w166, "SS.Telescope"=w160, "error"=w162) -> (w165:T16)
                n90 = Format Into String(format string="Error: %s", initial string=w163, w161) -> (resulting string=w159:string)  [unwired: 1 in, 1 out]
                n91 = call "CC System Message.vi"("Message"=w159) -> ()  [unwired: 10 in, 1 out]
              }
            }
          }
          frame "init detector" {
            n92 = Unbundle By Name(w181) -> ("Data Q"=w176:refnum<queue>, "SS.Detector"=w174:refnum<class "Detector.lvclass">, "Hardware.Installed Hardware"=w171:T6[])
            n93 = call "CC Get Current Device.vi"("Device Type Name"="detector", "Hardware.Installed Hardware"=w171) -> ("error out"=w169:errorcluster, "Curr Device Name"=w170:string)  [unwired: 7 in, 1 out]
            n94 = call-dynamic "SS Class Init.vi"("VI Refnum"=refnum<vi> refnum, "error in (no error)"=w169, "Device"=w170, "Detector in"=w174) -> ("error out"=w183:errorcluster, "Channel List"=w177:refnum<class "HK Item.lvclass">[], "Detector out"=w173:refnum<class "Detector.lvclass">)  [unwired: 5 in]
            n95 = call "SS Read vi ref.vi"("error in (no error)"=w183, "Subsystem Class in"=w173) -> ("error out"=w167:errorcluster, "vi ref"=w168:refnum<vi>, "Subsystem Class out"=w178:refnum<class "Detector.lvclass">)  [unwired: 7 in]
            n96 = Format Into String(format string="Initializing Detector %s.", w170) -> (resulting string=w179:string)  [unwired: 2 in, 1 out]
            n97 = invoke on="Detector Panel" class="SubPnl" method="Insert VI"(error in=w167, "VI Ref"=w168) -> ()  [unwired: 2 in, 4 out]
            n98 = case shown="Error .." w167 {
              selector: w167 -> [_ w197]
              tunnel: w179 -> [w184 w198]
              tunnel: w181 -> [w190 w201]
              tunnel: [w191 w200] -> w182
              tunnel: w178 -> [w193 w195]
              tunnel: w177 -> [w186 _]
              tunnel: w176 -> [w188 _]
              frame No Error {
                n99 = property class="Detector.lvclass"(reference=w193) -> (reference out=w189:refnum<class "Detector.lvclass">, "cmd q"=w192:T8)  [unwired: 1 in, 1 out]
                n100 = Bundle By Name(cluster=T17 {"Source"="Add Channels", "Type"="Command", "Data"=variant} ("element"), "Data"=w186) -> (w185:T17)
                n101 = call "CC System Message.vi"("Message"=w184) -> ()  [unwired: 10 in, 1 out]
                n102 = Enqueue Element(queue=w188, element=w185) -> ()  [unwired: 2 in, 3 out]
                n103 = Bundle By Name(cluster=w190, "SS.Detector"=w189, "Cmd Qs.Detector Q"=w192) -> (w191:T16)
              }
              frame Error {
                n104 = Unbundle By Name(w197) -> ("source"=w196:string)
                n105 = Bundle By Name(cluster=w201, "SS.Detector"=w195, "error"=w197) -> (w200:T16)
                n106 = Format Into String(format string="Error: %s", initial string=w198, w196) -> (resulting string=w194:string)  [unwired: 1 in, 1 out]
                n107 = call "CC System Message.vi"("Message"=w194) -> ()  [unwired: 10 in, 1 out]
              }
            }
          }
          frame "init temp control 1" {
            n108 = Unbundle By Name(w204) -> ("Data Q"=w206:refnum<queue>)  [unwired: 1 out]
            n109 = for {
              N: 1 -> [_]
              tunnel: w206 -> [w217]
              tunnel: "temp control" ("Device Type Name") -> [w214]
              shift-right: [w209] -> w203
              shift-left: w204 -> [w211]
              i -> [w213]
              n110 = Increment(x=w213) -> (x+1=w212:i32)
              n111 = Format Into String(format string=" %d", initial string=w214, w212) -> (resulting string=w207:string)  [unwired: 1 in, 1 out]
              n112 = call "SS Launch Subsystem.vi"("Curr Device Name"=w207, "Data Q"=w217) -> ("cmd q"=w208:T8, "vi ref"=w216:refnum<vi>, "Temp Ctl Class"=w210:refnum<class "Subsystem Class Temp Control.lvclass">)  [unwired: 6 in, 1 out]
              n113 = case shown="2" w213 {
                tunnel: w216 -> [w218 w223 w228]
                tunnel: w211 -> [w222 w227 w232]
                tunnel: w210 -> [w221 w226 w231]
                tunnel: [w220 w225 w230] -> w209
                tunnel: w208 -> [w219 w224 w229]
                frame 0, Default {
                  n114 = Bundle By Name(cluster=w222, "SS.Temp Ctl 1"=w221, "Cmd Qs.Temp Ctl 1"=w219) -> (w220:T16)
                  n115 = invoke on="Temp 1" class="SubPnl" method="Insert VI"("VI Ref"=w218) -> ()  [unwired: 3 in, 4 out]
                }
                frame 1 {
                  n116 = Bundle By Name(cluster=w227, "SS.Temp Ctl 2"=w226, "Cmd Qs.Temp Ctl 2"=w224) -> (w225:T16)
                  n117 = invoke on="Temp Ctl 2" class="SubPnl" method="Insert VI"("VI Ref"=w223) -> ()  [unwired: 3 in, 4 out]
                }
                frame 2 {
                  n118 = Bundle By Name(cluster=w232, "SS.Temp Ctl 3"=w231, "Cmd Qs.Temp Ctl 3"=w229) -> (w230:T16)
                  n119 = invoke on="Temp Ctl 3" class="SubPnl" method="Insert VI"("VI Ref"=w228) -> ()  [unwired: 3 in, 4 out]
                }
              }
            }
          }
          frame "init temp control 2", "init temp control 3" {
          }
          frame "init cryoserver" {
            n120 = Unbundle By Name(w244) -> ("SS.CryoServer"=w248:refnum<class "Subsystem CryoServer.lvclass">, "Hardware.Installed Hardware"=w237:T6[])
            n121 = call "CC Get Current Device.vi"("Device Type Name"="cryoserver", "Hardware.Installed Hardware"=w237) -> ("error out"=w235:errorcluster, "Curr Device Name"=w236:string)  [unwired: 7 in, 1 out]
            n122 = call-dynamic "SS Class Init.vi"("VI Refnum"=refnum<vi> refnum, "error in (no error)"=w235, "Device"=w236, "Subsystem CryoServer in"=w248) -> ("error out"=w246:errorcluster, "Subsystem CryoServer out"=w247:refnum<class "Subsystem CryoServer.lvclass">)  [unwired: 5 in, 1 out]
            n123 = call "SS Read vi ref.vi"("error in (no error)"=w246, "Subsystem Class in"=w247) -> ("error out"=w234:errorcluster, "vi ref"=w239:refnum<vi>, "Subsystem Class out"=w241:refnum<class "Subsystem CryoServer.lvclass">)  [unwired: 7 in]
            n124 = Format Into String(format string="Initializing CryoServer %s.", w236) -> (resulting string=w242:string)  [unwired: 2 in, 1 out]
            n125 = invoke on="Cryo Panel" class="SubPnl" method="Insert VI"("VI Ref"=w239) -> ()  [unwired: 3 in, 4 out]
            n126 = case shown="Error .." w234 {
              selector: w234 -> [_ w258]
              tunnel: w242 -> [w249 w259]
              tunnel: w244 -> [w251 w262]
              tunnel: [w252 w261] -> w245
              tunnel: w241 -> [w254 w256]
              frame No Error {
                # "Note: All Cryo Channels are dynamic\nso no add channels here."
                n127 = property class="Subsystem CryoServer.lvclass"(reference=w254) -> (reference out=w250:refnum<class "Subsystem CryoServer.lvclass">, "cmd q"=w253:T8)  [unwired: 1 in, 1 out]
                n128 = call "CC System Message.vi"("Message"=w249) -> ()  [unwired: 10 in, 1 out]
                n129 = Bundle By Name(cluster=w251, "SS.CryoServer"=w250, "Cmd Qs.CryoServer Q"=w253) -> (w252:T16)
              }
              frame Error {
                n130 = Unbundle By Name(w258) -> ("source"=w257:string)
                n131 = Bundle By Name(cluster=w262, "SS.CryoServer"=w256, "error"=w258) -> (w261:T16)
                n132 = Format Into String(format string="Error: %s", initial string=w259, w257) -> (resulting string=w255:string)  [unwired: 1 in, 1 out]
                n133 = call "CC System Message.vi"("Message"=w255) -> ()  [unwired: 10 in, 1 out]
              }
            }
          }
          frame "init focus" {
            n134 = Unbundle By Name(w276) -> ("SS.Focus"=w269:refnum<class "Subsystem Class Focus.lvclass">, "Hardware.Installed Hardware"=w271:T6[])
            n135 = call "CC Get Current Device.vi"("Device Type Name"="focus", "Hardware.Installed Hardware"=w271) -> ("error out"=w266:errorcluster, "Curr Device Name"=w267:string)  [unwired: 7 in, 1 out]
            n136 = call-dynamic "SS Class Init.vi"("VI Refnum"=refnum<vi> refnum, "error in (no error)"=w266, "Device"=w267, "Subsystem Class Focus in"=w269) -> ("error out"=w264:errorcluster, "Subsystem Class Focus out"=w265:refnum<class "Subsystem Class Focus.lvclass">)  [unwired: 5 in, 1 out]
            n137 = call "SS Read vi ref.vi"("error in (no error)"=w264, "Subsystem Class in"=w265) -> ("error out"=w263:errorcluster, "vi ref"=w270:refnum<vi>, "Subsystem Class out"=w273:refnum<class "Subsystem Class Focus.lvclass">)  [unwired: 7 in]
            n138 = Format Into String(format string="Initializing Focus System %s.", w267) -> (resulting string=w274:string)  [unwired: 2 in, 1 out]
            n139 = invoke on="Focus Panel" class="SubPnl" method="Insert VI"(error in=w263, "VI Ref"=w270) -> ()  [unwired: 2 in, 4 out]
            n140 = case shown="No Error" w263 {
              selector: w263 -> [_ w287]
              tunnel: w274 -> [w279 w288]
              tunnel: w276 -> [w281 w291]
              tunnel: [w282 w290] -> w277
              tunnel: w273 -> [w283 w285]
              frame No Error {
                n141 = property class="Subsystem Class Focus.lvclass"(reference=w283) -> (reference out=w280:refnum<class "Subsystem Class Focus.lvclass">, "cmd q"=w278:T8)  [unwired: 1 in, 1 out]
                n142 = call "CC System Message.vi"("Message"=w279) -> ()  [unwired: 10 in, 1 out]
                n143 = Bundle By Name(cluster=w281, "SS.Focus"=w280, "Cmd Qs.Focus Q"=w278) -> (w282:T16)
              }
              frame Error {
                n144 = Unbundle By Name(w287) -> ("source"=w286:string)
                n145 = Bundle By Name(cluster=w291, "SS.Focus"=w285, "error"=w287) -> (w290:T16)
                n146 = Format Into String(format string="Error: %s", initial string=w288, w286) -> (resulting string=w284:string)  [unwired: 1 in, 1 out]
                n147 = call "CC System Message.vi"("Message"=w284) -> ()  [unwired: 10 in, 1 out]
              }
            }
          }
          frame "init cryocooler" {
            n148 = Unbundle By Name(w307) -> ("Data Q"=w292:refnum<queue>, "SS.CryoCooler"=w301:refnum<class "Subsystem CryoCooler.lvclass">, "Hardware.Installed Hardware"=w302:T6[])
            n149 = call "CC Get Current Device.vi"("Device Type Name"="cryocooler", "Hardware.Installed Hardware"=w302) -> ("error out"=w298:errorcluster, "Curr Device Name"=w299:string)  [unwired: 7 in, 1 out]
            n150 = call-dynamic "SS Class Init.vi"("VI Refnum"=refnum<vi> refnum, "error in (no error)"=w298, "Device"=w299, "Subsystem CryoCooler in"=w301) -> ("error out"=w296:errorcluster, "Channel List"=w293:refnum<class "HK Item.lvclass">[], "Subsystem CryoCooler out"=w297:refnum<class "Subsystem CryoCooler.lvclass">)  [unwired: 5 in]
            n151 = call "SS Read vi ref.vi"("error in (no error)"=w296, "Subsystem Class in"=w297) -> ("error out"=w295:errorcluster, "vi ref"=w294:refnum<vi>, "Subsystem Class out"=w304:refnum<class "Subsystem CryoCooler.lvclass">)  [unwired: 7 in]
            n152 = Format Into String(format string="Initializing CryoCooler System %s.", w299) -> (resulting string=w305:string)  [unwired: 2 in, 1 out]
            n153 = invoke on="Telescope Panel" class="SubPnl" method="Insert VI"("VI Ref"=w294) -> ()  [unwired: 3 in, 4 out]
            n154 = case shown="No Error" w295 {
              selector: w295 -> [_ w322]
              tunnel: w305 -> [w314 w323]
              tunnel: w307 -> [w316 w326]
              tunnel: [w317 w325] -> w308
              tunnel: w304 -> [w318 w320]
              tunnel: w293 -> [w310 _]
              tunnel: w292 -> [w309 _]
              frame No Error {
                n155 = property class="Subsystem CryoCooler.lvclass"(reference=w318) -> (reference out=w315:refnum<class "Subsystem CryoCooler.lvclass">, "cmd q"=w313:T8)  [unwired: 1 in, 1 out]
                n156 = Bundle By Name(cluster=T17 {"Source"="Add Channels", "Type"="Command", "Data"=variant} ("element"), "Data"=w310) -> (w311:T17)
                n157 = call "CC System Message.vi"("Message"=w314) -> ()  [unwired: 10 in, 1 out]
                n158 = Bundle By Name(cluster=w316, "SS.CryoCooler"=w315, "Cmd Qs.CryoCooler Q"=w313) -> (w317:T16)
                n159 = Enqueue Element(queue=w309, element=w311) -> ()  [unwired: 2 in, 3 out]
              }
              frame Error {
                n160 = Unbundle By Name(w322) -> ("source"=w321:string)
                n161 = Bundle By Name(cluster=w326, "SS.CryoCooler"=w320, "error"=w322) -> (w325:T16)
                n162 = Format Into String(format string="Error: %s", initial string=w323, w321) -> (resulting string=w319:string)  [unwired: 1 in, 1 out]
                n163 = call "CC System Message.vi"("Message"=w319) -> ()  [unwired: 10 in, 1 out]
              }
            }
          }
          frame "init pressure monitor" {
            n164 = Unbundle By Name(w342) -> ("Data Q"=w328:refnum<queue>, "SS.Pressure"=w336:refnum<class "Subsystem Pressure Monitor.lvclass">, "Hardware.Installed Hardware"=w337:T6[])
            n165 = call "CC Get Current Device.vi"("Device Type Name"="pressure monitor", "Hardware.Installed Hardware"=w337) -> ("error out"=w333:errorcluster, "Curr Device Name"=w334:string)  [unwired: 7 in, 1 out]
            n166 = call-dynamic "SS Class Init.vi"("VI Refnum"=refnum<vi> refnum, "error in (no error)"=w333, "Device"=w334, "Subsystem Pressure Monitor in"=w336) -> ("error out"=w331:errorcluster, "Channel List"=w329:refnum<class "HK Item.lvclass">[], "Subsystem Pressure Monitor out"=w332:refnum<class "Subsystem Pressure Monitor.lvclass">)  [unwired: 5 in]
            n167 = call "SS Read vi ref.vi"("error in (no error)"=w331, "Subsystem Class in"=w332) -> ("error out"=w330:errorcluster, "vi ref"=w327:refnum<vi>, "Subsystem Class out"=w339:refnum<class "Subsystem Pressure Monitor.lvclass">)  [unwired: 7 in]
            n168 = Format Into String(format string="Initializing Pressure Monitor  System %s.", w334) -> (resulting string=w340:string)  [unwired: 2 in, 1 out]
            n169 = invoke on="Pressure Panel" class="SubPnl" method="Insert VI"("VI Ref"=w327) -> ()  [unwired: 3 in, 4 out]
            n170 = case shown="No Error" w330 {
              selector: w330 -> [_ w357]
              tunnel: w340 -> [w349 w358]
              tunnel: w342 -> [w351 w361]
              tunnel: [w352 w360] -> w343
              tunnel: w339 -> [w353 w355]
              tunnel: w329 -> [w345 _]
              tunnel: w328 -> [w344 _]
              frame No Error {
                n171 = property class="Subsystem Pressure Monitor.lvcl"(reference=w353) -> (reference out=w350:refnum<class "Subsystem Pressure Monitor.lvclass">, "cmd q"=w348:T8)  [unwired: 1 in, 1 out]
                n172 = Bundle By Name(cluster=T17 {"Source"="Add Channels", "Type"="Command", "Data"=variant} ("element"), "Data"=w345) -> (w346:T17)
                n173 = call "CC System Message.vi"("Message"=w349) -> ()  [unwired: 10 in, 1 out]
                n174 = Bundle By Name(cluster=w351, "SS.Pressure"=w350, "Cmd Qs.Pressure Q"=w348) -> (w352:T16)
                n175 = Enqueue Element(queue=w344, element=w346) -> ()  [unwired: 2 in, 3 out]
              }
              frame Error {
                n176 = Unbundle By Name(w357) -> ("source"=w356:string)
                n177 = Bundle By Name(cluster=w361, "SS.Pressure"=w355, "error"=w357) -> (w360:T16)
                n178 = Format Into String(format string="Error: %s", initial string=w358, w356) -> (resulting string=w354:string)  [unwired: 1 in, 1 out]
                n179 = call "CC System Message.vi"("Message"=w354) -> ()  [unwired: 10 in, 1 out]
              }
            }
          }
          frame "init scripting" {
            n180 = Unbundle By Name(w364) -> ("Cmd Qs"=w367:T7)
            n181 = vi-ref "CC Script GUI.vi"() -> (w376:refnum<vi>)
            n182 = Obtain Queue(name (unnamed)="Script Queue", element data type=T19 {"Cmd"="", "Parameters"=variant}) -> (queue out=w368:refnum<queue>)  [unwired: 3 in, 2 out]
            n183 = property class="VI (strict)"(reference=w376) -> (error out=w377:errorcluster, "Path"=w375:path)  [unwired: 1 in, 1 out]
            n184 = Bundle By Name(cluster=w367, "Script Q"=w368) -> (w366:T7)
            n185 = Open VI Reference(type specifier VI Refnum (for type only)=w376, vi path=w375, options=128, error in (no error)=w377) -> (vi reference=w374:refnum<vi>, error out=w372:errorcluster)  [unwired: 2 in]
            n186 = call-by-ref "Start Asynchronous Call"(reference=w374, error in=w372, "Standalone"=FALSE, "Cmd Qs"=w366) -> (error out=w371:errorcluster)  [unwired: 10 in, 1 out]
            n187 = Bundle By Name(cluster=w364, "Cmd Qs"=w366) -> (w365:T16)
            n188 = invoke on="Scripting Panel" class="SubPnl" method="Insert VI"(error in=w371, "VI Ref"=w376) -> (error out=w362:errorcluster)  [unwired: 2 in, 3 out]
            n189 = call <vilib>:"Clear Errors.vi"("error in (no error)"=w362) -> ()  [unwired: 5 in, 2 out]
          }
          frame "init observation list" {
            n190 = call "CC Get Filter Names.vi"() -> ("Wheel names"=w384:string[], "filter names"=w386:cluster{"Names":string[]}[])  [unwired: 9 in, 1 out]
            n191 = Unbundle By Name(w395) -> ("System Settings.Obs File"=w388:path, "state"=w394:refnum<user-event>, "Wheel Ref"=w385:refnum<vi>[])
            n192 = vi-ref "CC Observation Queue GUI.vi"() -> (w389:refnum<vi>)
            n193 = for {
              tunnel: w386 -> [w403] mode=indexing
              tunnel: w385 -> [w402] mode=indexing
              tunnel: w384 -> [w400] mode=indexing
              n194 = Unbundle(w403) -> ("Names"=w401:string[])
              n195 = property on="Property Node" class="Ring (strict)"(reference=w402, "Strings []"=w401, "Caption.Text"=w400) -> ()  [unwired: 1 in, 2 out]
            }
            n196 = property class="VI (strict)"(reference=w389) -> (error out=w392:errorcluster, "Path"=w391:path)  [unwired: 1 in, 1 out]
            n197 = Empty String/Path?(string/path=w388) -> (empty?=w381:bool)
            n198 = Open VI Reference(type specifier VI Refnum (for type only)=w389, vi path=w391, options=128, error in (no error)=w392) -> (vi reference=w380:refnum<vi>, error out=w378:errorcluster)  [unwired: 2 in]
            n199 = case shown="False" w381 {
              tunnel: [w399 _] -> w397
              tunnel: w388 -> [w398 _]
              frame False {
                n200 = call "CC Rd Wr Observation List.vi"("filepath"=w398) -> ("Observation List"=w399:T10[])  [unwired: 7 in, 3 out]
              }
              frame True {
              }
            }
            n201 = call-by-ref "Start Asynchronous Call"(reference=w380, error in=w378) -> (reference out=w379:refnum<vi>)  [unwired: 12 in, 1 out]
            n202 = Generate User Event(user event=w394, event data cluster="show observation" ("event data")) -> (error out=w382:errorcluster)  [unwired: 2 in, 1 out]
            n203 = call "CC create observation queue.vi"() -> ("Observation Queue"=w393:refnum<queue>)  [unwired: 10 in, 1 out]
            n204 = property on="Observation List" class="MCListbox (strict)"(error in=w382, "Val(Sgnl)"=i32[] [0] ("Value (Signaling)")) -> ()  [unwired: 1 in, 2 out]
            n205 = invoke on="Sub Panel" class="SubPnl" method="Insert VI"("VI Ref"=w379) -> ()  [unwired: 3 in, 4 out]
            n206 = Bundle By Name(cluster=w395, "Queue vi ref"=w379, "Obs Queue"=w393, "Observation List"=w397, "System Settings.Obs File"=w388) -> (w396:T16)
          }
          frame "load observation file" {
            n207 = call "CC Rd Wr Observation List.vi"() -> ("file"=w407:path, "Observation List"=w408:T10[])  [unwired: 8 in, 2 out]
            n208 = Unbundle By Name(w404) -> ("state"=w406:refnum<user-event>)
            n209 = Empty Array?(array=w408) -> (empty?=w409:bool)
            n210 = case shown="False" w409 {
              tunnel: w404 -> [w415 w416]
              tunnel: w408 -> [w414 _]
              tunnel: w407 -> [w413 _]
              tunnel: [w412 w416] -> w405
              tunnel: w406 -> [w411 _]
              frame False {
                n211 = Bundle By Name(cluster=w415, "Observation List"=w414, "System Settings.Obs File"=w413) -> (w412:T16)
                n212 = Generate User Event(user event=w411, event data cluster="show observation" ("event data")) -> ()  [unwired: 2 in, 2 out]
              }
              frame True {
              }
            }
          }
          frame "save observation file" {
            n213 = Unbundle By Name(w419) -> ("Observation List"=w420:T10[], "System Settings.Obs File"=w417:path)
            n214 = Strip Path(path=w417) -> (stripped path=w425:path, name=w426:string)
            n215 = call "File Dialog4"("start path"=w425, "default name"=w426, "pattern (all files)"="*.csv") -> ("selected path"=w421:path, "cancelled"=w422:bool, "error out"=w423:errorcluster)  [unwired: 9 in, 1 out]
            n216 = call <vilib>:"Clear Errors.vi"("error in (no error)"=w423) -> ()  [unwired: 5 in, 2 out]
            n217 = case shown="False" w422 {
              tunnel: w421 -> [w428 _]
              tunnel: w420 -> [w432 _]
              tunnel: w419 -> [w429 w433]
              tunnel: [w430 w433] -> w418
              frame False {
                n218 = Strip Path(path=w428) -> (name=w427:string)  [unwired: 1 out]
                n219 = call "CC Rd Wr Observation List.vi"("filepath"=w428, "Write? (F:Read)"=TRUE, "Observation List"=w432) -> ()  [unwired: 5 in, 4 out]
                n220 = local write "Observation File"(w427) -> ()
                n221 = Bundle By Name(cluster=w429, "System Settings.Obs File"=w428) -> (w430:T16)
              }
              frame True {
              }
            }
          }
          frame "save observation" {
            n222 = Unbundle By Name(w437) -> ("Observation List"=w436:T10[], "System Settings.Obs File"=w435:path)
            n223 = Empty String/Path?(string/path=w435) -> (empty?=w434:bool)
            n224 = case shown="False" w434 {
              tunnel: w436 -> [w439 _]
              tunnel: w435 -> [w438 _]
              frame False {
                n225 = call "CC Rd Wr Observation List.vi"("filepath"=w438, "Write? (F:Read)"=TRUE, "Observation List"=w439) -> ()  [unwired: 5 in, 4 out]
              }
              frame True {
              }
            }
          }
          frame "show observation" {
            n226 = Unbundle By Name(w446) -> ("Observation List"=w445:T10[], "System Settings.Obs File"=w442:path)
            n227 = call "CC Observation List to Table.vi"("Observation List"=w445) -> ("Screen Ready Table"=w443:string[][])  [unwired: 7 in, 3 out]
            n228 = Strip Path(path=w442) -> (name=→"Observation File":string)  [unwired: 1 out]
            n229 = call "CC Observation File Header.vi"() -> ("Header"=w444:string[])  [unwired: 10 in, 1 out]
            n230 = property on="Observation List" class="MCListbox (strict)"("ItemNames"=w443, "ColHdrString"=w444) -> ()  [unwired: 2 in, 2 out]
          }
          frame "show dithering" {
            n231 = local read "Dither"() -> (w449:T3)
            n232 = case shown="\"Random\"" w449 {
              tunnel: [T20."Disabled and Grayed Out" ("Disabled") T20."Enabled" ("Disabled") T20."Enabled" ("Disabled") T20."Enabled" ("Disabled")] -> w452
              tunnel: [FALSE TRUE TRUE FALSE] -> w451
              tunnel: [FALSE FALSE FALSE TRUE] -> w450
              tunnel: [FALSE TRUE FALSE FALSE] -> w448
              tunnel: [FALSE TRUE TRUE TRUE] -> w447
              frame "None" {
                n233 = property on="Spots" class="DigNum (strict)"("Value"=1 ("Spots")) -> ()  [unwired: 2 in, 2 out]
              }
              frame "Circle", Default {
              }
              frame "Random" {
              }
              frame "ABBA" {
                n234 = property on="Spots" class="DigNum (strict)"("Value"=4 ("Spots")) -> ()  [unwired: 2 in, 2 out]
              }
            }
            n235 = property on="Phase" class="DigNum (strict)"("Visible"=w448) -> ()  [unwired: 2 in, 2 out]
            n236 = property on="Radius" class="DigNum (strict)"("Visible"=w451) -> ()  [unwired: 2 in, 2 out]
            n237 = property on="RA Dither Offset" class="DigNum (strict)"("Visible"=w450) -> ()  [unwired: 2 in, 2 out]
            n238 = property on="Spots" class="DigNum (strict)"("Visible"=w447) -> ()  [unwired: 2 in, 2 out]
            n239 = property on="Spots" class="DigNum (strict)"("DisabledEnum"=w452) -> ()  [unwired: 2 in, 2 out]
            n240 = property on="DEC dither offset" class="DigNum (strict)"("Visible"=w450) -> ()  [unwired: 2 in, 2 out]
          }
          frame "generate script" {
            n241 = Unbundle By Name(w478) -> ("Cmd Qs.Script Q"=w481:T8, "System Settings.Obs File"=w477:path, "Observation List"=w491:T10[])
            n242 = call "Rd Wr Script Defaults.vi"() -> ("error out"=w480:errorcluster, "Script Settings"=w483:T29)  [unwired: 10 in]
            n243 = for {
              tunnel: w491 -> [w495] mode=indexing
              tunnel: [w494] -> w484 mode=concatenating
              shift-right: [w493] -> w479
              shift-left: w480 -> [w492]
              n244 = call "CC Observation to Script.vi"("error in (no error)"=w492, "Observation"=w495) -> ("error out"=w493:errorcluster, "Script Steps"=w494:T23[])  [unwired: 8 in]
            }
            n245 = call <vilib>:"Get File Extension.vi"("file"=w477) -> ("filename without extension"=w476:string)  [unwired: 6 in, 4 out]
            n246 = Unbundle By Name(w483) -> ("Script Path"=w482:path)
            n247 = call <vilib>:"Simple Error Handler.vi"("error in (no error)"=w479) -> ()  [unwired: 4 in, 5 out]
            n248 = Bundle By Name(cluster=T22 {"Name"="", "Script"=[]} ("Script"), "Name"=w476, "Script"=w484) -> (w489:T22)
            n249 = Bundle By Name(cluster=T19 {"Cmd"="", "Parameters"=variant} ("element"), "Cmd"="set script", "Parameters"=w476) -> (w486:T19)
            n250 = call "CC Rd Wr Script.vi"("Script Path"=w482, "Action"=CC_Rd_Wr_Script_Action."Write", "Script"=w489) -> ()  [unwired: 3 in, 6 out]
            n251 = Enqueue Element(queue=w481, element=w486) -> ()  [unwired: 2 in, 3 out]
          }
          frame "Check Alarms" {
            n252 = Unbundle By Name(w497) -> ("Cmd Qs.Script Q"=w499:T8, "alarm disable"=w496:bool, "Script Running"=w502:bool)
            n253 = call "CC Alarm Object.vi"("Alarm Action"=CC_enum_Alarm_Action."Get Alarms") -> ("Alarm List"=w514:T30[], "Alarm?"=w500:bool)  [unwired: 7 in, 2 out]
            "Alarm Status" <- w500
            n254 = Compound Arithmetic op=AND(invert w496, w502, w500) -> (w501:bool)
            n255 = for {
              tunnel: w514 -> [w530] mode=indexing
              tunnel: [w529] -> w513 mode=indexing
              tunnel: [w526] -> w504 mode=indexing
              n256 = Unbundle By Name(w530) -> ("Message"=w528:string, "Source"=w529:string)
              n257 = Concatenate Strings(w528, "\r\n") -> (w526:string)
            }
            n258 = case shown="True" w501 {
              tunnel: w499 -> [_ w521]
              tunnel: w497 -> [w516 w519]
              tunnel: [w516 w517] -> w498
              frame False {
              }
              frame True {
                n259 = Enqueue Element(queue=w521, element=T19 {"Cmd"="abort script", "Parameters"=variant}) -> ()  [unwired: 2 in, 3 out]
                n260 = Bundle By Name(cluster=w519, "Script Running"=FALSE) -> (w517:T16)
              }
            }
            n261 = for {
              tunnel: w513 -> [w525]
              tunnel: string[] ["Detector", "Filter Wheel", "Telescope", "Pressure Monitor", "CryoCooler", "CryoServer"] -> [w524] mode=indexing
              tunnel: [w522] -> w511 mode=indexing
              n262 = Search 1D Array(1D array=w525, element=w524) -> (index of element=w523:i32)  [unwired: 1 in]
              n263 = Greater Or Equal To 0?(x=w523) -> (x >= 0?=w522:bool)
            }
            n264 = Concatenate Strings(w504) -> (→"Alarm Message":string)
            n265 = Index Array(array=w511) -> (element #1=→"Detector Alarm":bool, element #2=→"FW Alarm":bool, element #3=→"Telescope Alarm":bool, element #4=→"Pressure Alarm":bool, element #5=→"Cryo Alarm":bool, element #6=→"Temp":bool)  [unwired: 6 in]
          }
          frame "Update Table" {
            n266 = call "Elapsed Time"() -> ("Time has Elapsed"=w539:bool)  [unwired: 12 in, 7 out]
            n267 = Unbundle By Name(w542) -> ("Data Q"=w540:refnum<queue>, "state"=w538:refnum<user-event>)
            n268 = call "CC Log Object.vi"("Action"=CC_enum_Current_Values_Action."Get Current Values") -> ("error out"=w546:errorcluster, "HK Channel out"=w537:refnum<class "HK Table.lvclass">)  [unwired: 8 in, 1 out]
            n269 = case shown="True" w539 {
              tunnel: w538 -> [_ w552]
              frame False {
              }
              frame True {
                n270 = Generate User Event(user event=w552, event data cluster="Show Plot" ("event data")) -> ()  [unwired: 2 in, 2 out]
              }
            }
            n271 = call "CC Past Noon Check.vi"() -> ("Passed noon"=w541:bool)  [unwired: 10 in, 1 out]
            n272 = call-dynamic "HK Channel Get Formatted Value Table.vi"("error in (no error)"=w546, "HK Table in"=w537) -> ("Hdr"=w544:string[], "Table"=w545:string[][])  [unwired: 5 in, 3 out]
            n273 = case shown="True" w541 {
              tunnel: w540 -> [_ w554]
              frame False {
              }
              frame True {
                n274 = Enqueue Element(queue=w554, element=T17 {"Source"="New File", "Type"="Command", "Data"=variant}) -> ()  [unwired: 2 in, 3 out]
              }
            }
            n275 = for {
              tunnel: w537 -> [w550]
              tunnel: string[] ["Telescope RA", "Telescope DEC"] -> [w549] mode=indexing
              tunnel: [w548] -> w535 mode=indexing
              tunnel: [w547] -> w531
              n276 = call-dynamic "HK Channel Read Formatted Value.vi"("Name"=w549, "HK Table.lvclass"=w550) -> ("error out"=w547:errorcluster, "Value"=w548:dbl)  [unwired: 2 in, 6 out]
            }
            n277 = property on="Channels" class="MCListbox (strict)"("ItemNames"=w545, "ColHdrString"=w544) -> ()  [unwired: 2 in, 2 out]
            n278 = Array To Cluster(array=w535) -> (cluster=w534:cluster{"[0]":dbl, "[1]":dbl})
            n279 = call <vilib>:"Clear Errors.vi"("error in (no error)"=w531) -> ()  [unwired: 5 in, 2 out]
            n280 = call "CC Convert RA and DEC to HHMMSS.vi"("RA and DEC"=w534) -> ("DEC String"=→"Current DEC":string, "RA String"=→"Current RA":string)  [unwired: 7 in, 2 out]
          }
          frame "Show Plot" {
            n281 = property on="Channels" class="MCListbox (strict)"() -> ("ItemNames"=w567:string[][])  [unwired: 2 in, 2 out]
            n282 = for {
              tunnel: w567 -> [w596]
              tunnel: "Channels" -> [w595] mode=indexing
              tunnel: [w593] -> w563 mode=indexing
              tunnel: [w592] -> w565 mode=indexing
              n283 = Index Array(array=w596, index (row)=w595, index (col)=3 ("disabled index (col)")) -> (element=w592:string)
              n284 = Index Array(array=w596, index (row)=w595, index (col)=0 ("disabled index (col)")) -> (element=w593:string)
            }
            n285 = call "CC Read Channels from TDMS File.vi"("Sources"=w565, "ItemNames"=w563) -> ("error out"=w562:errorcluster, "units"=w556:string[], "Y Axes"=w561:i32[], "XY Graph"=w564:cluster{timestamp[], dbl[]}[])  [unwired: 6 in]
            n286 = Array Size(array=w556) -> (size(s)=w555:i32)
            n287 = for {
              N: 3 -> [_]
              tunnel: [w572] -> w558
              tunnel: w555 -> [w570]
              i -> [w571]
              n288 = Less?(x=w571, y=w570) -> (x < y?=w569:bool)
              n289 = property on="XY Graph" class="XYGraph (strict)"("ActYScl"=w571, "YScale.Visible"=w569) -> (error out=w572:errorcluster)  [unwired: 2 in, 1 out]
            }
            n290 = flat-sequence {
              tunnel: w564 -> [w576]
              tunnel: w562 -> [w575]
              tunnel: w561 -> [w574]
              tunnel: [w574] -> w560
              tunnel: w556 -> [w573]
              tunnel: [w573] -> w559
              tunnel: w558 -> [_]
              tunnel: w563 -> [w582]
              tunnel: w560 -> [w581]
              tunnel: w559 -> [w580]
              frame #0 {
                n291 = call <vilib>:"Clear Errors.vi"("error in (no error)"=w575) -> ()  [unwired: 5 in, 2 out]
                "XY Graph" <- w576
              }
              frame #1 {
                n292 = for {
                  N: 3 -> [_]
                  tunnel: w580 -> [w585] mode=indexing
                  tunnel: [w583] -> w577
                  i -> [w586]
                  n293 = property on="XY Graph" class="XYGraph (strict)"("ActYScl"=w586, "YScale.NameLbl.Text"=w585, "YScale.Visible"=TRUE ("Y Scale.Visible")) -> (error out=w583:errorcluster)  [unwired: 2 in, 1 out]
                }
                n294 = for {
                  N -> [w589]
                  tunnel: w582 -> [w590] mode=indexing
                  tunnel: w581 -> [w588] mode=indexing
                  tunnel: [w587] -> w578
                  i -> [w591]
                  n295 = property on="XY Graph" class="XYGraph (strict)"("Active Plot"=w591, "Plot.Plot Name"=w590, "LegNumRows"=w589, "Plot.YScaleIdx"=w588) -> (error out=w587:errorcluster)  [unwired: 2 in, 1 out]
                }
                n296 = call <vilib>:"Clear Errors.vi"("error in (no error)"=w578) -> ()  [unwired: 5 in, 2 out]
                n297 = call <vilib>:"Clear Errors.vi"("error in (no error)"=w577) -> ()  [unwired: 5 in, 2 out]
              }
            }
          }
          frame "Script Status" {
            n298 = Unbundle By Name(w598) -> ("Status Data"=w608:variant)
            n299 = Variant To Data(type=T27 {"Time"=timestamp(0 s since 1904-01-01), "Running"=FALSE, "Step"=0, "Script Name"="", "Step Name"=""}, Variant=w608) -> (data=w607:T27)  [unwired: 1 in, 1 out]
            n300 = Unbundle By Name(w607) -> ("Step"=w605:i32, "Step Name"=w601:string, "Running"=w600:bool)
            n301 = Format Into String(format string="Step %d: %s", w605, w601) -> (resulting string=w604:string)  [unwired: 2 in, 1 out]
            n302 = Select(t=w604, s=w600, f="Idle") -> (s? t:f=→"Status":string)
            n303 = Bundle By Name(cluster=w598, "Script Running"=w600) -> (w599:T16)
          }
          frame "New Image", "Script New Images" {
            w613 = map{string, path} {}  # Size: 0
            n304 = call "CC FG Recent Images.vi"() -> ("Recent Images out"=w619:T31[])  [unwired: 10 in, 1 out]
            n305 = Index Array(array=w619) -> (element=w620:T31)  [unwired: 1 in]
            n306 = Unbundle By Name(w620) -> ("FITS file"=w612:path)
            n307 = Strip Path(path=w612) -> (stripped path=w611:path)  [unwired: 1 out]
            n308 = case shown="False" FALSE {
              tunnel: w619 -> [_ w642]
              tunnel: [w627 w641] -> w618
              tunnel: [w628 w640] -> w615
              tunnel: w613 -> [w629 w639]
              tunnel: w611 -> [w625 w638]
              tunnel: [w621 w638] -> w610
              frame False {
                w627 = string[] ["raw", "res"]
                n309 = Strip Path(path=w625) -> (stripped path=w626:path, name=w624:string)
                n310 = Strip Path(path=w626) -> (stripped path=w633:path)  [unwired: 1 out]
                n311 = Build Path(base path=w633, name or relative path=path "res") -> (appended path=w631:path)
                n312 = Build Path(base path=w631, name or relative path=w624) -> (appended path=w630:path)
                n313 = Build Array(w625, w630) -> (w623:path[])
                n314 = for {
                  shift-right: [w634] -> w628
                  shift-left: w629 -> [w637]
                  tunnel: w627 -> [w636] mode=indexing
                  tunnel: w623 -> [w635] mode=indexing
                  n315 = Insert Into Map(map in=w637, key=w636, value=w635) -> (map out=w634:map{string, path})  [unwired: 2 out]
                }
                n316 = property on="Image Type" class="Ring (strict)"() -> ("Value"=w622:u16)  [unwired: 2 in, 2 out]
                n317 = Index Array(array=w623, index=w622) -> (element=w621:path)
              }
              frame True {
                n318 = for {
                  tunnel: w642 -> [w650] mode=indexing
                  shift-right: [w647] -> w640
                  shift-left: w639 -> [w649]
                  n319 = Unbundle By Name(w650) -> ("Image Type"=w648:string, "FITS file"=w646:path)
                  n320 = Strip Path(path=w646) -> (stripped path=w645:path)  [unwired: 1 out]
                  n321 = Insert Into Map(map in=w649, key=w648, value=w645) -> (map out=w647:map{string, path})  [unwired: 2 out]
                }
                n322 = for {
                  tunnel: w640 -> [w644] mode=indexing
                  tunnel: [w643] -> w641 mode=indexing
                  n323 = Unbundle By Name(w644) -> ("type"=w643:string)
                }
              }
            }
            n324 = Bundle By Name(cluster=w616, "image types"=w615) -> (w617:T16)
            n325 = property on="Data Folder" class="Path"("Val(Sgnl)"=w610) -> ()  [unwired: 2 in, 2 out]
            n326 = property on="Image Type" class="Ring (strict)"("Strings []"=w618) -> ()  [unwired: 2 in, 2 out]
          }
          frame "Load Image Folder" {
            n327 = Unbundle By Name(w656) -> ("System Settings.Images Folder"=w654:path)
            n328 = disable-structure shown="Disabled" {
              disable-tunnel: w654 -> [w660 _]
              frame Disabled {
                n329 = control-ref of="Recent Images"() -> (w658:refnum<vi>)
                n330 = invoke on="Invoke Node" class="LstBox (strict)" method="Edit Tree Items.Delete"(reference=w658) -> (reference out=w657:refnum<vi>)  [unwired: 4 in, 4 out]
                n331 = call "CC GUI Recursive Load Folder to Tree.vi"("Tree Ref"=w657, "Depth"=3, "Path"=w660) -> ()  [unwired: 8 in, 1 out]
              }
              frame Enabled {
              }
            }
            n332 = List Folder(path=w654, pattern="*.fits") -> (filenames=w653:string[])  [unwired: 2 in, 3 out]
            n333 = call "Sort 1D Array.vim"("unsorted array"=w653) -> ("sorted array"=w652:string[])  [unwired: 10 in]
            n334 = Reverse 1D Array(array=w652) -> (reversed array=w651:string[])
            n335 = property on="Recent Images" class="LstBox (strict)"("Item Names"=w651) -> ()  [unwired: 2 in, 2 out]
          }
          frame "Load Image" {
            n336 = Unbundle By Name(w663) -> ("state"=w666:refnum<user-event>, "curr image"=w662:path)
            n337 = Generate User Event(user event=w666, event data cluster="Update Zoom" ("event data")) -> ()  [unwired: 2 in, 2 out]
            n338 = call "CC FITS Read Image.vi"("FITS File Path"=w662) -> ("Image"=w661:sgl[][])  [unwired: 9 in, 1 out]
            "Thumbnail" <- w661
            n339 = Bundle By Name(cluster=w663, "image"=w661) -> (w664:T16)
          }
          frame "generate observation" {
            n340 = control-ref of="Filter 1"() -> (w686:refnum<vi>)
            n341 = control-ref of="Filter 2"() -> (w685:refnum<vi>)
            n342 = control-ref of="Filter 3"() -> (w684:refnum<vi>)
            n343 = control-ref of="Filter 4"() -> (w683:refnum<vi>)
            n344 = Build Array(w686, w685, w684, w683) -> (w682:refnum<vi>[])
            n345 = call "CC Filter Names from Control Refs.vi"("Filter Refs"=w682) -> ("Filter names"=w681:string[])  [unwired: 9 in, 1 out]
            n346 = Format Into String("Obj Type") -> (resulting string=w673:string)  [unwired: 3 in, 1 out]
            n347 = call <vilib>:"Trim Whitespace.vi"("string"="Observer") -> ("trimmed string"=w672:string)  [unwired: 1 in]
            n348 = call <vilib>:"Trim Whitespace.vi"("string"=w673) -> ("trimmed string"=w671:string)  [unwired: 1 in]
            n349 = call <vilib>:"Trim Whitespace.vi"("string"="Obj Name") -> ("trimmed string"=w670:string)  [unwired: 1 in]
            n350 = call <vilib>:"Trim Whitespace.vi"("string"="RA") -> ("trimmed string"=w669:string)  [unwired: 1 in]
            n351 = call <vilib>:"Trim Whitespace.vi"("string"="DEC") -> ("trimmed string"=w668:string)  [unwired: 1 in]
            n352 = call <vilib>:"Trim Whitespace.vi"("string"="Comment") -> ("trimmed string"=w667:string)  [unwired: 1 in]
            n353 = Bundle By Name(cluster=T10 {"Priority"=0, "ID"="", "Observer"="", "Obj Name"="", "Obj Type"="", "RA and DEC String"={"RA"="12:34:56.789", "DEC"="010:11:12.013"}, "Filters"=[], "Integration Time"=0.0, "Observation Status"=enum."Ready", "Offsets"={"xi"=0.0, "eta"=0.0, "Offset Type"=enum."SIMPLE"}, "Images"=0, "Dither Options"={"Dither"=enum."None", "Dither Radius"=0.0, "Dither Points"=0, "Dither Phase"=0.0, "B Offset"={"RA"=0.0, "DEC"=0.0}}, "Comment 1"="", "Comment 2"="", "Rotator"={"Frame"=enum."Target", "PA"=0.0}} ("Observation"), "Observer"=w672, "Obj Type"=w671, "Obj Name"=w670, "RA and DEC String.RA"=w669, "RA and DEC String.DEC"=w668, "Filters"=w681, "Offsets.xi"="xi", "Offsets.eta"="eta", "Rotator.PA"="ROT PA", "Dither Options.Dither"="Dither", "Dither Options.Dither Phase"="Phase", "Dither Options.Dither Radius"="Radius", "Integration Time"="Int Time", "Dither Options.Dither Points"="Spots", "Images"="Images", "Priority"="Priority", "Comment 1"=w667, "Dither Options.B Offset.RA"="RA Dither Offset", "Dither Options.B Offset.DEC"="DEC dither offset") -> (w677:T10)
            n354 = Bundle By Name(cluster=w675, "Observation"=w677) -> (w676:T16)
          }
          frame "start quick image" {
            n355 = Unbundle By Name(w706) -> ("Obs Queue"=w705:refnum<queue>, "Observation"=w703:T10)
            n356 = Bundle By Name(cluster=T28 {"Msg"="quick image", "Data"=variant} ("element"), "Data"=w703) -> (w702:T28)
            n357 = Enqueue Element(queue=w705, element=w702) -> ()  [unwired: 2 in, 3 out]
          }
          frame "inject observation" {
            n358 = Unbundle By Name(w713) -> ("Obs Queue"=w712:refnum<queue>, "Observation"=w709:T10)
            n359 = Bundle By Name(cluster=w709, "Observation Status"=CC_enum_Observation_Status."Ready") -> (w708:T10)
            n360 = Bundle By Name(cluster=T28 {"Msg"="addtop", "Data"=variant} ("element"), "Data"=w708) -> (w711:T28)
            n361 = Enqueue Element(queue=w712, element=w711) -> ()  [unwired: 2 in, 3 out]
          }
          frame "replace observation" {
            n362 = Unbundle By Name(w721) -> ("Observation List"=w715:T10[], "Observation"=w719:T10)
            n363 = local read "Observation List"() -> (w724:i32[])
            n364 = call "CC Observation Check For BlockID.vi"("Generate ID?"=TRUE, "BlockID"="Block ID", "Observation List"=w715) -> ("BlockID string"=w714:string)  [unwired: 6 in, 2 out]
            n365 = Index Array(array=w724) -> (element=w720:i32)  [unwired: 1 in]
            n366 = Bundle By Name(cluster=w719, "ID"=w714) -> (w718:T10)
            n367 = Replace Array Subset(array=w715, new element=w718, index=w720) -> (w723:T10[])
            n368 = Bundle By Name(cluster=w721, "Observation List"=w723) -> (w722:T16)
          }
          frame "add observation" {
            n369 = Unbundle By Name(w725) -> ("Observation List"=w730:T10[], "Observation"=w729:T10)
            n370 = call "CC Next ID.vi"() -> ("BlockID string"=w731:string)  [unwired: 9 in, 2 out]
            n371 = Bundle By Name(cluster=w729, "ID"=w731) -> (w728:T10)
            n372 = Build Array (concatenate)(w730, w728) -> (w727:T10[])
            n373 = Bundle By Name(cluster=w725, "Observation List"=w727) -> (w726:T16)
          }
          frame "Update Zoom" {
            w751 = 0.19
            # "plate scale"
            # "slit"
            # "star"
            n374 = property on="Thumbnail" class="IntGraph (strict)"() -> ("Cursor.Cursor Y"=w769:dbl, "Cursor.Cursor X"=w767:dbl, "CrsrLis"=w758:T32, "ZScale.Maximum"=w744:dbl, "ZScale.Minimum"=w743:dbl, "XScale.Maximum"=w742:dbl, "XScale.Minimum"=w739:dbl, "YScale.Maximum"=w741:dbl, "YScale.Minimum"=w738:dbl)  [unwired: 2 in, 2 out]
            n375 = property on="Waveform Graph" class="WFGraph (strict)"("ActYScl"=0, "YScale.Maximum"=w744, "YScale.Minimum"=w743) -> ()  [unwired: 2 in, 2 out]
            n376 = property on="Waveform Graph" class="WFGraph (strict)"("ActYScl"=1, "YScale.Maximum"=w744, "YScale.Minimum"=w743) -> ()  [unwired: 2 in, 2 out]
            n377 = Index Array(array=w758, index=1) -> (element=w756:T33)
            n378 = Index Array(array=w758, index=0) -> (element=w757:T33)
            n379 = Unbundle By Name(w770) -> ("image"=w768:sgl[][])
            n380 = Divide(x="zoom size", y=2) -> (x/y=w734:dbl)
            n381 = Subtract(x=w769, y=w734) -> (x-y=w761:dbl)
            n382 = Subtract(x=w767, y=w734) -> (x-y=w760:dbl)
            n383 = Array Subset(array=w768, index (row)=w761, length (row)="zoom size", index (col)=w760, length (col)="zoom size") -> (→"Zoom":sgl[][])
            n384 = Index Array(array=w768, index (col)=w767) -> (element=w765:sgl[])  [unwired: 1 in]
            n385 = Index Array(array=w768, index (row)=w769) -> (element=w766:sgl[])  [unwired: 1 in]
            n386 = Unbundle By Name(w757) -> ("Position.X"=w733:dbl)
            n387 = Unbundle By Name(w756) -> ("Position.Y"=w754:dbl)
            n388 = Unbundle By Name(w756) -> ("Position.X"=w732:dbl)
            n389 = Unbundle By Name(w757) -> ("Position.Y"=w755:dbl)
            n390 = Max & Min(x=w742, y=w741) -> (max(x,y)=w740:dbl)  [unwired: 1 out]
            n391 = Max & Min(x=w739, y=w738) -> (min(x,y)=w737:dbl)  [unwired: 1 out]
            n392 = Bundle("image"=w766) -> (w764:cluster{"image":sgl[]})  [unwired: 1 in]
            n393 = Bundle("image"=w765) -> (w763:cluster{"image":sgl[]})  [unwired: 1 in]
            n394 = Build Array(w764, w763) -> (→"Waveform Graph":cluster{"image":sgl[]}[])
            n395 = property on="Waveform Graph" class="WFGraph (strict)"("XScale.Maximum"=w740, "XScale.Minimum"=w737) -> ()  [unwired: 2 in, 2 out]
            n396 = Subtract(x=w732, y=w733) -> (x-y=w753:dbl)
            n397 = Subtract(x=w755, y=w754) -> (x-y=w752:dbl)
            n398 = Multiply(x=w753, y=w751) -> (x*y=w750:dbl)
            n399 = Multiply(x=w752, y=w751) -> (x*y=w749:dbl)
            n400 = Build Array(w750, w749) -> (→"offset (\")":dbl[])
          }
          frame "Shutdown" {
            n401 = Unbundle By Name(w773) -> ("state"=w779:refnum<user-event>, "System Settings"=w775:T9)
            n402 = call "CC System Message.vi"("Message"="System Shutdown Starting") -> ()  [unwired: 10 in, 1 out]
            n403 = Generate User Event(user event=w779, event data cluster="shutdown subsystems" ("event data")) -> (user event out=w778:refnum<user-event>)  [unwired: 2 in, 1 out]
            n404 = call "Rd Wr System Settings.vi"("Write? (F:Read)"=TRUE, "System Settings"=w775) -> ()  [unwired: 8 in, 2 out]
            n405 = Generate User Event(user event=w778, event data cluster="shutdown all" ("event data")) -> ()  [unwired: 2 in, 2 out]
          }
          frame "shutdown subsystems" {
            n406 = Unbundle By Name(w782) -> ("SS"=w781:T34)
            n407 = Cluster To Array(cluster=w781) -> (array=w780:refnum<class "Subsystem Class.lvclass">[])
            n408 = for {
              tunnel: w780 -> [w784] mode=indexing
              n409 = call-dynamic "SS Close.vi"("Subsystem Class in"=w784) -> ("error out"=w785:errorcluster)  [unwired: 9 in, 1 out]
              n410 = call <vilib>:"Clear Errors.vi"("error in (no error)"=w785) -> ()  [unwired: 5 in, 2 out]
            }
          }
          frame "shutdown all" {
            # "Empty array to plot memory"
            n411 = Unbundle By Name(w792) -> ("Quad Viewer Ref"=w789:refnum<vi>, "Viewer Ref"=w790:refnum<vi>, "Cmd Qs.Script Q"=w794:T8, "Data Q"=w797:refnum<queue>, "Obs Queue"=w787:refnum<queue>)
            n412 = Enqueue Element(queue=w787, element=T28 {"Msg"="shutdown", "Data"=variant}) -> ()  [unwired: 2 in, 3 out]
            n413 = Build Array(w789, w790) -> (w788:refnum<vi>[])
            n414 = for {
              tunnel: w788 -> [w798] mode=indexing
              n415 = invoke class="VI" method="Abort VI"(reference=w798) -> (reference out=w800:refnum<vi>, error out=w801:errorcluster)  [unwired: 2 in, 1 out]
              n416 = Close Reference(reference=w800, error in (no error)=w801) -> (error out=w799:errorcluster)
              n417 = call <vilib>:"Clear Errors.vi"("error in (no error)"=w799) -> ()  [unwired: 5 in, 2 out]
            }
            n418 = Enqueue Element(queue=w797, element=T17 {"Source"="Shutdown", "Type"="Command", "Data"=variant}) -> ()  [unwired: 2 in, 3 out]
            n419 = Enqueue Element(queue=w794, element=T19 {"Cmd"="Shutdown", "Parameters"=variant}) -> ()  [unwired: 2 in, 3 out]
            n420 = local write "Thumbnail"(sgl[][] [] ("Thumbnail")) -> ()
          }
        }
      }
      event "Add offsets": Value Change {
        n421 = event-data() -> ()  [unwired: 1 in, 6 out]
        n422 = local read "offset (\")"() -> (w808:dbl[])
        n423 = property on="xi" class="DigNum (strict)"() -> ("Value"=w805:dbl)  [unwired: 2 in, 2 out]
        n424 = property on="eta" class="DigNum (strict)"() -> ("Value"=w804:dbl)  [unwired: 2 in, 2 out]
        n425 = Index Array(array=w808) -> (element #1=w807:dbl, element #2=w806:dbl)  [unwired: 2 in]
        n426 = Add(x=w804, y=w806) -> (x+y=w802:dbl)
        n427 = Add(x=w805, y=w807) -> (x+y=w803:dbl)
        n428 = property on="xi" class="DigNum (strict)"("Val(Sgnl)"=w803) -> ()  [unwired: 2 in, 2 out]
        n429 = property on="eta" class="DigNum (strict)"("Val(Sgnl)"=w802) -> ()  [unwired: 2 in, 2 out]
      }
      event Menu Selection (User) {
        n430 = event-data() -> ("MenuRef"=w810:refnum<k9>, "ItemTag"=w813:string)  [unwired: 1 in, 1 out]
        n431 = case shown="\"Select Hardware\"" w813 {
          selector: w813 -> [w816 _ _ _ _ _ _ w872 _]
          tunnel: w812 -> [w814 w818 w819 w831 w843 w848 w852 w867 w875]
          tunnel: [w814 w818 w819 w828 w843 w848 w850 w865 w875] -> w811
          tunnel: w810 -> [_ _ _ _ _ _ _ w874 _]
          frame "True", Default {
            n432 = Format Into String(format string="Main Menu Item %s not implemented.", w816) -> (resulting string=w815:string)  [unwired: 2 in, 1 out]
            n433 = One Button Dialog(message=w815) -> ()  [unwired: 1 in, 1 out]
          }
          frame "Edit FITS Header" {
            n434 = call "CC FITS Make FITS Header Table.vi"() -> ()  [unwired: 12 in]
          }
          frame "Restore Previous Setup" {
            n435 = Unbundle By Name(w819) -> ("state"=w821:refnum<user-event>)
            n436 = call "CC Restore Previous Setup.vi"() -> ("Select File"=w820:path, "Restored?"=w822:bool)  [unwired: 10 in]
            n437 = case shown="True" w822 {
              tunnel: w821 -> [_ w827]
              tunnel: w820 -> [_ w824]
              frame False {
              }
              frame True {
                n438 = Generate User Event(user event=w827, event data cluster="Shutdown" ("event data")) -> ()  [unwired: 2 in, 2 out]
                n439 = Format Into String(format string="User restored setup file from config archive. Restored to %s. System shutting down for restart.", w824) -> (resulting string=w823:string)  [unwired: 2 in, 1 out]
                n440 = call "CC System Message.vi"("Message"=w823) -> ()  [unwired: 10 in, 1 out]
              }
            }
          }
          frame "Select Hardware" {
            n441 = Unbundle By Name(w831) -> ("state"=w830:refnum<user-event>, "Hardware"=w834:T5)
            n442 = call "CC Hardware Config Dialog.vi"() -> ("Hardware Config"=w832:T5)  [unwired: 11 in]
            n443 = Not Equal?(x=w834, y=w832) -> (x != y?=w833:bool)
            n444 = case shown="True" w833 {
              tunnel: w832 -> [_ w839]
              tunnel: w831 -> [w835 w840]
              tunnel: w830 -> [_ w838]
              tunnel: string[] ["shutdown subsystems", "init subsystems"] -> [_ w837]
              tunnel: [w835 w836] -> w828
              frame False {
              }
              frame True {
                n445 = for {
                  tunnel: w838 -> [w842]
                  tunnel: w837 -> [w841] mode=indexing
                  n446 = Generate User Event(user event=w842, event data cluster=w841) -> ()  [unwired: 2 in, 2 out]
                }
                n447 = Bundle By Name(cluster=w840, "Hardware"=w839) -> (w836:T16)
              }
            }
          }
          frame "Load Observation File" {
            n448 = Unbundle By Name(w843) -> ("state"=w845:refnum<user-event>)
            n449 = Generate User Event(user event=w845, event data cluster="load observation file" ("event data")) -> ()  [unwired: 2 in, 2 out]
          }
          frame "Save Observation File as..." {
            n450 = Unbundle By Name(w848) -> ("state"=w846:refnum<user-event>)
            n451 = Generate User Event(user event=w846, event data cluster="save observation file" ("event data")) -> ()  [unwired: 2 in, 2 out]
          }
          frame "New Observation File" {
            n452 = Unbundle By Name(w852) -> ("state"=w849:refnum<user-event>, "System Settings.Obs File"=w857:path)
            n453 = Strip Path(path=w857) -> (stripped path=w856:path)  [unwired: 1 out]
            n454 = call "File Dialog3"("start path"=w856, "default name"="New Observation", "pattern (all files)"="*.csv") -> ("selected path"=w851:path, "cancelled"=w853:bool)  [unwired: 9 in, 2 out]
            n455 = case shown="False" w853 {
              tunnel: w852 -> [w863 w864]
              tunnel: w851 -> [w861 _]
              tunnel: [w860 w864] -> w850
              tunnel: w849 -> [w858 _]
              frame False {
                n456 = Bundle By Name(cluster=w863, "System Settings.Obs File"=w861, "Observation List"=T10[] []) -> (w860:T16)
                n457 = Generate User Event(user event=w858, event data cluster="show observation" ("event data")) -> ()  [unwired: 2 in, 2 out]
              }
              frame True {
              }
            }
          }
          frame "Disable Alarms" {
            n458 = Get Menu Item Info(7:w872, 11:w874) -> (0:w870:errorcluster, 1:w868:bool, 2:w869:string, 3:w873:refnum<k9>, 4:w871:bool)  [unwired: 1 in, 2 out]
            n459 = Not(x=w871) -> (.not. x?=w866:bool)
            n460 = Set Menu Item Info(6:w866, 7:w872, 8:w870, 9:w868, 10:w869, 11:w873) -> ()  [unwired: 1 in, 2 out]
            n461 = Bundle By Name(cluster=w867, "alarm disable"=w866) -> (w865:T16)
          }
          frame "Exit" {
            n462 = Unbundle By Name(w875) -> ("state"=w877:refnum<user-event>)
            n463 = Generate User Event(user event=w877, event data cluster="Shutdown" ("event data")) -> ()  [unwired: 2 in, 2 out]
          }
        }
      }
      event "Load": Value Change {
        n464 = event-data() -> ()  [unwired: 1 in, 6 out]
        n465 = Unbundle By Name(w878) -> ("state"=w880:refnum<user-event>)
        n466 = Generate User Event(user event=w880, event data cluster="load observation file" ("event data")) -> ()  [unwired: 2 in, 2 out]
      }
      event "Save As Button": Value Change {
        n467 = event-data() -> ()  [unwired: 1 in, 6 out]
        n468 = Unbundle By Name(w881) -> ("state"=w883:refnum<user-event>)
        n469 = Generate User Event(user event=w883, event data cluster="save observation file" ("event data")) -> ()  [unwired: 2 in, 2 out]
      }
      event "Observation List": Value Change {
        n470 = event-data() -> ()  [unwired: 1 in, 1 out]
        n471 = Unbundle By Name(w917) -> ("state"=w890:refnum<user-event>, "Observation List"=w916:T10[])
        n472 = Index Array(array="Observation List") -> (element=w905:i32)  [unwired: 1 in]
        n473 = Index Array(array=w916, index=w905) -> (element=w914:T10)
        n474 = Generate User Event(user event=w890, event data cluster="show dithering" ("event data")) -> ()  [unwired: 2 in, 2 out]
        n475 = property on="Obj Type" class="Enum (strict)"() -> ("Strings []"=w886:string[])  [unwired: 2 in, 2 out]
        n476 = Unbundle By Name(w914) -> ("Priority"=w898:i32, "ID"=w904:string, "Observer"=w913:string, "Obj Name"=w912:string, "RA and DEC String.RA"=w911:string, "RA and DEC String.DEC"=w910:string, "Filters"=w892:string[], "Dither Options.Dither"=w909:T3, "Dither Options.Dither Radius"=w908:dbl, "Integration Time"=w907:dbl, "Dither Options.Dither Points"=w906:i32, "Images"=w903:i32, "Dither Options.Dither Phase"=w902:dbl, "Offsets.xi"=w901:dbl, "Offsets.eta"=w900:dbl, "Rotator.PA"=w899:dbl, "Comment 1"=w897:string, "Dither Options.B Offset.RA"=w888:dbl, "Dither Options.B Offset.DEC"=w887:dbl, "Obj Type"=w885:string)
        n477 = local write "RA Dither Offset"(w888) -> ()
        n478 = local write "DEC dither offset"(w887) -> ()
        n479 = Search 1D Array(1D array=w886, element=w885) -> (index of element=w884:i32)  [unwired: 1 in]
        n480 = local write "Obj Name"(w912) -> ()
        n481 = local write "Observer"(w913) -> ()
        n482 = local write "Block ID"(w904) -> ()
        n483 = local write "Priority"(w898) -> ()
        n484 = local write "DEC"(w910) -> ()
        n485 = local write "RA"(w911) -> ()
        n486 = control-ref of="Filter 1"() -> (w896:refnum<vi>)
        n487 = control-ref of="Filter 2"() -> (w895:refnum<vi>)
        n488 = control-ref of="Filter 3"() -> (w894:refnum<vi>)
        n489 = control-ref of="Filter 4"() -> (w893:refnum<vi>)
        n490 = local write "Obj Type"(w884) -> ()
        n491 = Build Array(w896, w895, w894, w893) -> (w891:refnum<vi>[])
        n492 = local write "Comment"(w897) -> ()
        n493 = local write "ROT PA"(w899) -> ()
        n494 = local write "Int Time"(w907) -> ()
        n495 = local write "Images"(w903) -> ()
        n496 = local write "Radius"(w908) -> ()
        n497 = local write "eta"(w900) -> ()
        n498 = local write "Dither"(w909) -> ()
        n499 = local write "Phase"(w902) -> ()
        n500 = local write "Spots"(w906) -> ()
        n501 = local write "xi"(w901) -> ()
        n502 = call "CC Set Filter Strings.vi"("Strings"=w892, "refs"=w891) -> ()  [unwired: 9 in, 1 out]
      }
      event "Observation List": Shortcut Menu Activation? {
        n503 = event-data() -> ()  [unwired: 1 in, 7 out]
        n504 = event-data("Discard?"=FALSE) -> ()  [unwired: 1 in, 1 out]
      }
      event "Observation List": Shortcut Menu Selection (User) {
        n505 = event-data() -> ("ItemTag"=w929:string, "CtlRef"=w931:refnum<vi>, "Coords"=w930:T35)  [unwired: 1 in]
        n506 = invoke class="MCListbox (strict)" method="Point To Row Column"(reference=w931, "Point"=w930) -> ("CellPosition"=w927:T36)  [unwired: 5 in, 6 out]
        n507 = Unbundle By Name(w924) -> ("Observation List"=w928:T10[])
        n508 = Unbundle By Name(w924) -> ("state"=w923:refnum<user-event>)
        n509 = case shown="\"Send to Bottom of Queue\"" w929 {
          tunnel: w928 -> [w932 w936 w941 w947]
          tunnel: w927 -> [_ w935 w942 w948]
          tunnel: [w932 w933 w937 w943] -> w925
          frame "False", Default {
          }
          frame "Delete Item" {
            n510 = Unbundle By Name(w935) -> ("Row"=w934:i32)
            n511 = Delete From Array(array=w936, index=w934) -> (array with subset deleted=w933:T10[])  [unwired: 1 in, 1 out]
          }
          frame "Send to Top of Queue" {
            n512 = Unbundle By Name(w942) -> ("Row"=w940:i32)
            n513 = Delete From Array(array=w941, index=w940) -> (deleted portion=w939:T10, array with subset deleted=w938:T10[])  [unwired: 1 in]
            n514 = Build Array (concatenate)(w939, w938) -> (w937:T10[])
          }
          frame "Send to Bottom of Queue" {
            n515 = Unbundle By Name(w948) -> ("Row"=w946:i32)
            n516 = Delete From Array(array=w947, index=w946) -> (deleted portion=w945:T10, array with subset deleted=w944:T10[])  [unwired: 1 in]
            n517 = Build Array (concatenate)(w944, w945) -> (w943:T10[])
          }
        }
        n518 = Generate User Event(user event=w923, event data cluster="show observation" ("event data")) -> (user event out=w921:refnum<user-event>)  [unwired: 2 in, 1 out]
        n519 = Generate User Event(user event=w921, event data cluster="save observation" ("event data")) -> ()  [unwired: 2 in, 2 out]
        n520 = Bundle By Name(cluster=w924, "Observation List"=w925) -> (w926:T16)
      }
      event "Add to Q", "Add to Q top": Value Change {
        n521 = event-data() -> ()  [unwired: 1 in, 6 out]
        n522 = Unbundle By Name(w954) -> ("Obs Queue"=w951:refnum<queue>, "Observation List"=w953:T10[])
        n523 = local read "Observation List"() -> (w952:i32[])
        n524 = for {
          tunnel: w953 -> [w969]
          tunnel: w952 -> [w968] mode=indexing
          tunnel: w951 -> [w967]
          tunnel: "Add to Q" -> [w965]
          tunnel: CC_enum_Observation_Status."Ready" ("Observation Status") -> [w955]
          n525 = Index Array(array=w969, index=w968) -> (element=w958:T10)
          n526 = Bundle By Name(cluster=w958, "Observation Status"=w955) -> (w956:T10)
          n527 = Select(t=T28 {"Msg"="addend", "Data"=variant} ("element"), s=w965, f=T28 {"Msg"="addtop", "Data"=variant} ("element")) -> (s? t:f=w960:T28)
          n528 = Bundle By Name(cluster=w960, "Data"=w958) -> (w966:T28)
          n529 = Unbundle By Name(w956) -> ("ID"=w957:string)
          n530 = Unbundle By Name(w960) -> ("Msg"=w959:string)
          n531 = Enqueue Element(queue=w967, element=w966) -> ()  [unwired: 2 in, 3 out]
          n532 = Format Into String(format string="Sending observation %s to queue with command %s. ", w957, w959) -> (resulting string=w962:string)  [unwired: 2 in, 1 out]
          n533 = call "CC System Message.vi"("Message"=w962) -> ()  [unwired: 10 in, 1 out]
        }
      }
      event "Generate Script": Value Change {
        n534 = event-data() -> ()  [unwired: 1 in, 6 out]
        n535 = Unbundle By Name(w985) -> ("Cmd Qs.Script Q"=w973:T8, "System Settings.Obs File"=w972:path, "Observation List"=w984:T10[])
        n536 = call "Rd Wr Script Defaults.vi"() -> ("error out"=w971:errorcluster, "Script Settings"=w975:T29)  [unwired: 10 in]
        n537 = for {
          tunnel: w984 -> [w989] mode=indexing
          tunnel: [w988] -> w976 mode=concatenating
          shift-right: [w987] -> w970
          shift-left: w971 -> [w986]
          n538 = call "CC Observation to Script.vi"("error in (no error)"=w986, "Observation"=w989) -> ("error out"=w987:errorcluster, "Script Steps"=w988:T23[])  [unwired: 8 in]
        }
        n539 = Unbundle By Name(w975) -> ("Script Path"=w974:path)
        n540 = Strip Path(path=w972) -> (name=w977:string)  [unwired: 1 out]
        n541 = call <vilib>:"Simple Error Handler.vi"("error in (no error)"=w970) -> ()  [unwired: 4 in, 5 out]
        n542 = Bundle By Name(cluster=T22 {"Name"="", "Script"=[]} ("Script"), "Name"=w977, "Script"=w976) -> (w982:T22)
        n543 = Bundle By Name(cluster=T19 {"Cmd"="", "Parameters"=variant} ("element"), "Cmd"="set script", "Parameters"=w977) -> (w979:T19)
        n544 = call "CC Rd Wr Script.vi"("Script Path"=w974, "Action"=CC_Rd_Wr_Script_Action."Write", "Script"=w982) -> ()  [unwired: 3 in, 6 out]
        n545 = Enqueue Element(queue=w973, element=w979) -> ()  [unwired: 2 in, 3 out]
      }
      event "Save Obs List": Value Change {
        n546 = event-data() -> ()  [unwired: 1 in, 6 out]
        n547 = Unbundle By Name(w991) -> ("System Settings.Obs File"=w999:path)
        n548 = Strip Path(path=w999) -> (stripped path=w997:path, name=w998:string)
        n549 = call "File Dialog"("start path"=w997, "default name"=w998, "pattern (all files)"="*.csv") -> ("selected path"=w994:path, "cancelled"=w995:bool, "error out"=w990:errorcluster)  [unwired: 9 in, 1 out]
        n550 = call <vilib>:"Clear Errors.vi"("error in (no error)"=w990) -> ()  [unwired: 5 in, 2 out]
        n551 = Unbundle By Name(w991) -> ("Observation List"=w993:T10[])
        n552 = case shown="False" w995 {
          tunnel: w994 -> [w1001 _]
          tunnel: w993 -> [w1004 _]
          tunnel: w991 -> [w1002 w1005]
          tunnel: [w1000 w1005] -> w992
          frame False {
            n553 = call "CC Rd Wr Observation List.vi"("filepath"=w1001, "Write? (F:Read)"=TRUE, "Observation List"=w1004) -> ()  [unwired: 5 in, 4 out]
            n554 = Bundle By Name(cluster=w1002, "System Settings.Obs File"=w1001) -> (w1000:T16)
          }
          frame True {
          }
        }
      }
      event "Add Obs Row", "Replace": Value Change {
        n555 = event-data() -> ("CtlRef"=w1014:refnum<vi>)  [unwired: 1 in]
        n556 = property class="Bool"(reference=w1014) -> ("Label.Text"=w1013:string)  [unwired: 1 in, 2 out]
        n557 = Equal?(x=w1013, y="Replace") -> (x = y?=w1010:bool)
        n558 = Unbundle By Name(w1011) -> ("state"=w1006:refnum<user-event>)
        n559 = Select(t=string[] ["generate observation", "replace observation", "show observation", "save observation"], s=w1010, f=string[] ["generate observation", "add observation", "show observation", "save observation"]) -> (s? t:f=w1007:string[])
        n560 = for {
          tunnel: w1007 -> [w1015] mode=indexing
          tunnel: w1006 -> [w1016]
          n561 = Generate User Event(user event=w1016, event data cluster=w1015) -> ()  [unwired: 2 in, 2 out]
        }
      }
      event Value Change {
        n562 = event-data() -> ()  [unwired: 1 in, 6 out]
        n563 = Unbundle By Name(w1019) -> ("state"=w1018:refnum<user-event>)
        n564 = Generate User Event(user event=w1018, event data cluster="show dithering" ("event data")) -> ()  [unwired: 2 in, 2 out]
      }
      event "RA": Value Change {
        n565 = event-data() -> ("NewVal"=w1021:string)  [unwired: 1 in, 5 out]
        n566 = call "CC Parse Right Ascension.vi"("Right Ascension string"=w1021) -> ("error out"=w1020:errorcluster)  [unwired: 8 in, 2 out]
        n567 = case shown="No Error" w1020 {
          selector: w1020 -> [_ w1024]
          frame No Error {
          }
          frame Error {
            n568 = Unbundle By Name(w1024) -> ("source"=w1023:string)
            n569 = One Button Dialog(message=w1023) -> ()  [unwired: 1 in, 1 out]
          }
        }
      }
      event "DEC": Value Change {
        n570 = event-data() -> ("NewVal"=w1026:string)  [unwired: 1 in]
        n571 = call "CC Parse Declination.vi"("Declination string"=w1026) -> ("error out"=w1025:errorcluster)  [unwired: 8 in, 2 out]
        n572 = case shown="Error .." w1025 {
          selector: w1025 -> [_ w1029]
          frame No Error {
          }
          frame Error {
            n573 = Unbundle By Name(w1029) -> ("source"=w1028:string)
            n574 = One Button Dialog(message=w1028) -> ()  [unwired: 1 in, 1 out]
          }
        }
      }
      event "Log", "Log 2": Value Change {
        n575 = event-data() -> ()  [unwired: 1 in, 6 out]
        n576 = Build Array("Log", "Log 2") -> (w1030:bool[])
        n577 = for {
          tunnel: w1030 -> [w1035] mode=indexing
          i -> [w1036]
          n578 = Boolean To (0,1)(Boolean=w1035) -> (0, 1=w1034:i16)
          n579 = property on="XY Graph" class="XYGraph (strict)"("ActYScl"=w1036, "YScale.Mapping Mode"=w1034) -> ()  [unwired: 2 in, 2 out]
        }
      }
      event "XY Graph": Mouse Enter {
        n580 = event-data() -> ("CtlRef"=w1038:refnum<vi>)  [unwired: 1 in]
        n581 = property class="XYGraph (strict)"(reference=w1038, "Legend Visible"=TRUE ("Legend:Visible")) -> ()  [unwired: 1 in, 2 out]
      }
      event "XY Graph": Mouse Leave {
        n582 = event-data() -> ("CtlRef"=w1041:refnum<vi>)  [unwired: 1 in]
        n583 = property class="XYGraph (strict)"(reference=w1041, "Legend Visible"=FALSE ("Legend:Visible")) -> ()  [unwired: 1 in, 2 out]
      }
      event "Channels": Value Change {
        n584 = event-data() -> ()  [unwired: 1 in, 6 out]
        n585 = Unbundle By Name(w1044) -> ("state"=w1043:refnum<user-event>)
        n586 = Generate User Event(user event=w1043, event data cluster="Show Plot" ("event data")) -> ()  [unwired: 2 in, 2 out]
      }
      event "Recent Images": Value Change {
        n587 = event-data() -> ("CtlRef"=w1050:refnum<vi>, "NewVal"=w1048:i32)  [unwired: 1 in, 1 out]
        n588 = Unbundle By Name(w1051) -> ("state"=w1054:refnum<user-event>, "System Settings.Images Folder"=w1046:path)
        n589 = property class="LstBox (strict)"(reference=w1050) -> ("Item Names"=w1049:string[])  [unwired: 1 in, 2 out]
        n590 = Index Array(array=w1049, index=w1048) -> (element=w1047:string)
        n591 = xnode "Match Regular Expression"("input string"=w1047, "regular expression"="(.*\\.fits)") -> ("submatch 1"=w1053:string)  [unwired: 4 in, 5 out]
        n592 = Empty String/Path?(string/path=w1053) -> (empty?=w1055:bool)
        n593 = case shown="False" w1055 {
          tunnel: w1054 -> [w1063 _]
          tunnel: w1053 -> [w1059 _]
          tunnel: w1051 -> [w1061 w1064]
          tunnel: [w1060 w1064] -> w1052
          tunnel: w1046 -> [w1058 _]
          frame False {
            n594 = Build Path(base path=w1058, name or relative path=w1059) -> (appended path=w1057:path)
            n595 = Generate User Event(user event=w1063, event data cluster="Load Image" ("event data")) -> ()  [unwired: 2 in, 2 out]
            n596 = Bundle By Name(cluster=w1061, "curr image"=w1057) -> (w1060:T16)
            "Current File" <- w1059
          }
          frame True {
          }
        }
      }
      event "Recent Images": Shortcut Menu Activation? {
        n597 = event-data() -> ("MenuRef"=w1192:refnum<k9>, "CtlRef"=w1186:refnum<vi>, "Coords"=w1185:T35)  [unwired: 1 in]
        n598 = property class="LstBox (strict)" props=["Item Names", "Value"](reference=w1186) -> ("Item Names"=w1191:string[])  [unwired: 1 in, 3 out]
        n599 = invoke class="LstBox (strict)" method="Point To Row"(reference=w1186, "Point"=w1185) -> ("Row"=w1184:i32)  [unwired: 5 in, 6 out]
        n600 = Unbundle By Name(w1189) -> ("System Settings.Images Folder"=w1188:path)
        n601 = Index Array(array=w1191, index=w1184) -> (element=w1190:string)
        n602 = Build Path(base path=w1188, name or relative path=w1190) -> (appended path=w1187:path)
        n603 = call <vilib>:"Check if File or Folder Exists.vi"("path"=w1187) -> ("file or folder exists?"=w1194:bool)  [unwired: 8 in, 2 out]
        n604 = Set Menu Item Info(7:"Explore..." ("item tag"), 9:w1194, 10:w1190, 11:w1192) -> ()  [unwired: 3 in, 2 out]
        n605 = event-data("Discard?"=FALSE) -> ()  [unwired: 1 in, 1 out]
      }
      event "Recent Images": Shortcut Menu Selection (User) {
        n606 = event-data() -> ("ItemTag"=w1205:string, "CtlRef"=w1198:refnum<vi>, "Coords"=w1197:T35)  [unwired: 1 in]
        n607 = Unbundle By Name(w1202) -> ("System Settings.Images Folder"=w1200:path)
        n608 = property class="LstBox (strict)"(reference=w1198) -> ("Item Names"=w1203:string[])  [unwired: 1 in, 2 out]
        n609 = invoke class="LstBox (strict)" method="Point To Row"(reference=w1198, "Point"=w1197) -> ("Row"=w1196:i32)  [unwired: 5 in, 6 out]
        n610 = Index Array(array=w1203, index=w1196) -> (element=w1201:string)
        n611 = Build Path(base path=w1200, name or relative path=w1201) -> (appended path=w1199:path)
        n612 = case shown="\"Open in Quad Viewer\"" w1205 {
          tunnel: w1202 -> [w1206 w1208 w1215]
          tunnel: [w1206 w1208 w1213] -> w1204
          tunnel: w1199 -> [_ w1207 w1212]
          frame "False", Default {
          }
          frame "Explore..." {
            n613 = call <vilib>:"Check if File or Folder Exists.vi"("path"=w1207) -> ("file or folder exists?"=w1210:bool, "dup path"=w1209:path)  [unwired: 8 in, 1 out]
            n614 = case shown="True" w1210 {
              tunnel: w1209 -> [_ w1211]
              frame False {
              }
              frame True {
                n615 = call <vilib>:"Show in File System.vi"("file or directory path"=w1211) -> ()  [unwired: 10 in, 1 out]
              }
            }
          }
          frame "Open in Quad Viewer" {
            # "Add quad viwer"
            n616 = call "CC Get All Files for Image.vi"("path"=w1212) -> ("Files for image"=w1216:path[])  [unwired: 9 in, 1 out]
            n617 = call "CC Launch Quad Viewer.vi"("Files"=w1216) -> ("reference out"=w1214:refnum<vi>)  [unwired: 9 in, 1 out]
            n618 = Bundle By Name(cluster=w1215, "Quad Viewer Ref"=w1214) -> (w1213:T16)
          }
        }
      }
      event "Thumbnail": Cursor Move; "zoom size": Value Change; "Thumbnail": Scale Range Change {
        n619 = event-data() -> ()  [unwired: 1 in, 4 out]
        n620 = Unbundle By Name(w1219) -> ("state"=w1218:refnum<user-event>)
        n621 = Generate User Event(user event=w1218, event data cluster="Update Zoom" ("event data")) -> ()  [unwired: 2 in, 2 out]
      }
      event "Waveform Graph": Mouse Enter {
        n622 = event-data() -> ("CtlRef"=w1221:refnum<vi>)  [unwired: 1 in]
        n623 = property class="WFGraph (strict)"(reference=w1221, "Legend Visible"=TRUE ("Legend:Visible")) -> ()  [unwired: 1 in, 2 out]
      }
      event "Waveform Graph": Mouse Leave {
        n624 = event-data() -> ("CtlRef"=w1223:refnum<vi>)  [unwired: 1 in]
        n625 = property class="WFGraph (strict)"(reference=w1223, "Legend Visible"=FALSE ("Legend:Visible")) -> ()  [unwired: 1 in, 2 out]
      }
      event "Send": Value Change {
        n626 = event-data() -> ()  [unwired: 1 in, 6 out]
        n627 = call "CC System Message.vi"("Message"="Note for Log") -> ()  [unwired: 10 in, 1 out]
      }
      event "Get Image": Value Change {
        (unwired) string[] ["generate observation", "start quick image"]
        n628 = event-data() -> ()  [unwired: 1 in, 6 out]
        n629 = Unbundle By Name(w1230) -> ("state"=w1229:refnum<user-event>)
        n630 = for {
          tunnel: w1229 -> [w1232]
          tunnel: string[] ["generate observation", "add observation", "show observation", "save observation", "inject observation"] -> [w1231] mode=indexing
          n631 = Generate User Event(user event=w1232, event data cluster=w1231) -> ()  [unwired: 2 in, 2 out]
        }
      }
      event "Close": Value Change; Panel Close {
        n632 = event-data() -> ()  [unwired: 1 in, 3 out]
        n633 = Unbundle By Name(w1236) -> ("state"=w1235:refnum<user-event>)
        n634 = Generate User Event(user event=w1235, event data cluster="Shutdown" ("event data")) -> ()  [unwired: 2 in, 2 out]
      }
      event "Tab Control": Value Change {
        n635 = event-data() -> ()  [unwired: 1 in, 6 out]
      }
      event "Open Log": Value Change {
        n636 = event-data() -> ()  [unwired: 1 in, 1 out]
        n637 = Unbundle By Name(w1245) -> ("file path"=w1244:path, "Viewer Ref"=w1239:refnum<vi>)
        n638 = Not A Number/Path/Refnum?(number/path/refnum=w1239) -> ()  [unwired: 1 out]
        n639 = Empty String/Path?(string/path=w1244) -> (empty?=w1243:bool)
        n640 = call "CC Log Object.vi"("Action"=CC_enum_Current_Values_Action."Get Current Values") -> ("Current File"=w1242:path)  [unwired: 8 in, 2 out]
        n641 = Select(t=w1242, s=w1243, f=w1244) -> (s? t:f=w1240:path)
        n642 = case shown="True" TRUE {
          tunnel: w1245 -> [w1247 w1258]
          tunnel: [w1247 w1257] -> w1241
          tunnel: w1240 -> [_ w1251]
          tunnel: w1239 -> [w1249 _]
          frame False {
            n643 = property class="VI Interface Type 0"(reference=w1249, "Front Panel.IsFrontmost"=TRUE ("Front Panel Window:Is Frontmost")) -> ()  [unwired: 1 in, 2 out]
          }
          frame True {
            n644 = vi-ref "NI_TDMS File Viewer.lvlib:TDMS - File Viewer (NXG Style).vi"() -> (w1256:refnum<vi>)
            n645 = property class="VI Interface Type 0"(reference=w1256) -> (reference out=w1253:refnum<vi>, "Path"=w1255:path)  [unwired: 1 in, 1 out]
            n646 = Open VI Reference(type specifier VI Refnum (for type only)=w1253, vi path=w1255, options=128) -> (vi reference=w1252:refnum<vi>)  [unwired: 3 in, 1 out]
            n647 = call-by-ref "Start Asynchronous Call"(reference=w1252, "file in"=w1251) -> (reference out=w1250:refnum<vi>)  [unwired: 10 in, 3 out]
            n648 = Bundle By Name(cluster=w1258, "Viewer Ref"=w1250) -> (w1257:T16)
          }
        }
      }
      event "Edit FITS Hdr": Value Change {
        n649 = event-data() -> ()  [unwired: 1 in, 6 out]
        n650 = call "CC FITS Make FITS Header Table.vi"() -> ()  [unwired: 12 in]
      }
      event "Clear Alarms": Value Change {
        n651 = event-data() -> ()  [unwired: 1 in, 6 out]
        n652 = Unbundle By Name(w1263) -> ("state"=w1262:refnum<user-event>)
        n653 = Generate User Event(user event=w1262, event data cluster="Check Alarms" ("event data")) -> ()  [unwired: 2 in, 2 out]
        n654 = call "CC Alarm Object.vi"("Alarm Action"=CC_enum_Alarm_Action."Clear All Alarms") -> ()  [unwired: 7 in, 4 out]
        n655 = call "CC System Message.vi"("Message"="User Cleared Alarm Manually") -> ()  [unwired: 10 in, 1 out]
      }
      event "Data Folder": Value Change {
        n656 = event-data() -> ()  [unwired: 1 in, 6 out]
        n657 = Unbundle By Name(w1270) -> ("state"=w1269:refnum<user-event>)
        n658 = Generate User Event(user event=w1269, event data cluster="Load Image Folder" ("event data")) -> ()  [unwired: 2 in, 2 out]
        n659 = Bundle By Name(cluster=w1270, "System Settings.Images Folder"="Data Folder") -> (w1267:T16)
        n660 = Unbundle By Name(w1267) -> ("System Settings"=w1266:T9)
        n661 = call "Rd Wr System Settings.vi"("Write? (F:Read)"=TRUE, "System Settings"=w1266) -> ()  [unwired: 8 in, 2 out]
      }
      event "Image Type": Value Change {
        n662 = event-data() -> ("CtlRef"=w1279:refnum<vi>)  [unwired: 1 in, 5 out]
        n663 = Unbundle By Name(w1276) -> ("image types"=w1275:map{string, path})
        n664 = property class="Ring (strict)"(reference=w1279) -> ("Strings []"=w1278:string[])  [unwired: 1 in, 2 out]
        n665 = Index Array(array=w1278, index="Image Type") -> (element=w1274:string)
        n666 = Look In Map(map=w1275, key=w1274) -> (key not found?=w1273:bool, value=w1272:path)  [unwired: 1 in]
        n667 = case shown="False" w1273 {
          tunnel: w1272 -> [w1280 _]
          frame False {
            n668 = property on="Data Folder" class="Path"("Val(Sgnl)"=w1280) -> ()  [unwired: 2 in, 2 out]
          }
          frame True {
          }
        }
      }
    }
  }
  n669 = Unbundle By Name(w7) -> ("Application:Kind"=w4:T4)
  n670 = Not Equal?(x=T4."Evaluation" ("y"), y=w4) -> (x != y?=w1:bool)
  n671 = Not Equal?(x=w4, y=T4."Development System") -> (x != y?=w5:bool)
  n672 = And(x=w1, y=w5) -> (x .and. y?=w2:bool)
  n673 = Quit LabVIEW(quit? (T)=w2) -> ()
